vi "Autonomous Independent.vi"() -> ()   [LabVIEW 2016]
doc: "This VI is called when autonomous begins, and will automatically be terminated when autonomous ends. You can carry out timed or sensor driven robot movement independently without needing to return to the caller."
uses:
  <vilib>/Rock Robotics/WPI/ThirdParty/CanMotor/TalonSRX/WPI_CANTalonSRX_APIFeedbackSelect.ctl
  <vilib>/Rock Robotics/WPI/ThirdParty/CanMotor/TalonSRX/WPI_CANTalonSRX_Params.ctl
  <vilib>/Rock Robotics/WPI/ThirdParty/CanMotor/TalonSRX/WPI_CANTalonSRX_APIControlMode.ctl
  <vilib>/Rock Robotics/WPI/Utilities/WPI_GetSetVariantRefNum.vi
  <vilib>/Rock Robotics/Network Tables/NT Read String.vi
  <vilib>/Rock Robotics/Network Tables/NT Write Numeric Array.vi
  <vilib>/Rock Robotics/WPI/RobotDrive/WPI_RobotDriveArcadeDrive_Standard(NoSaturation).vi
  Robot Global Data.vi
panel:
  out "Encoder Position 7":dbl
  out "Encoder Position 6":dbl
  out "RIGHT SIDE":dbl
  out "Encoder Position 4":dbl
  out "Encoder Position 3":dbl
  out "Encoder Position":dbl
  out "Encoder Position 2":dbl
  # "Be sure to right-click and choose Data Operations>>Make Current Value default if you want to save the array values with the VI"
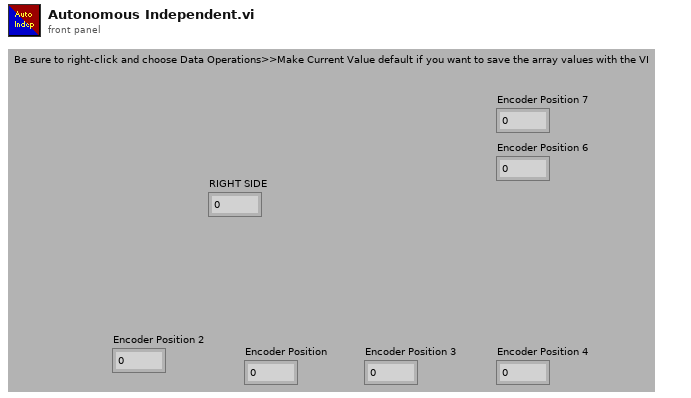
[diagram p1: front panel]
types:
  T1 = typedef "WPI_CANTalonSRX_APIFeedbackSelect.ctl" = enum16{"Digital Quadrature Encoder", "Analog Potentiometer", "Analog Encoder", "Count on Quad-A (Rising-Edge)", "Count on Quad-A (Falling-Edge)", "CTR Magnetic Enc (Absolute)", "CTR Magnetic Enc (Relative)", "Pulse Width"}
  T2 = typedef "WPI_JoystickDevRef.ctl" = cluster{"Device":T3}
  T3 = typedef "WPI_JoystickDeviceEnum.ctl" = enum16{"USB 0", "USB 1", "USB 2", "USB 3", "USB 4", "USB 5"}
  T4 = typedef "WPI_MotorControlDeviceRef.ctl" = cluster{"DeviceStatus":errorcluster, "Type":T5, "PWM":cluster{"PWM Channel":T6, "DeadBand":T7}, "CAN":cluster{"Device Number":u8, "SetOutput VI Ref":variant, "GetOutput VI Ref":variant, "Enable VI Ref":variant, "Disable VI Ref":variant, "Data":variant}, "Invert":bool}
  T5 = typedef "WPI_MotorControlType.ctl" = enum16{"PWM", "CAN"}
  T6 = typedef "FPGA_DIOPWMChannel.ctl" = enum8{"PWM 0", "PWM 1", "PWM 2", "PWM 3", "PWM 4", "PWM 5", "PWM 6", "PWM 7", "PWM 8", "PWM 9", "PWM MXP 0", "PWM MXP 1", "PWM MXP 2", "PWM MXP 3", "PWM MXP 4", "PWM MXP 5", "PWM MXP 6", "PWM MXP 7", "PWM MXP 8", "PWM MXP 9", "Invalid"}
  T7 = typedef "WPI_PWMDeadband.ctl" = cluster{"Name":string, "maxPositivePwm":i32, "minPositivePwm":i32, "centerPwm":i32, "maxNegativePwm":i32, "minNegativePwm":i32, "angularRange":u16}
  T8 = typedef "WPI_RobotDriveDevRef.ctl" = cluster{"DevStatus":errorcluster, "Motors[]":T4[], "Square Inputs":bool, "Max Output":dbl}
  T9 = typedef "WPI_CANTalonSRX_APIControlMode.ctl" = enum8{"Percent VBus", "Speed", "Position", "Slave", "Unchanged / Invalid", "Voltage Compensation", "Current", "Motion Profile", "Motion Magic"}
  T10 = typedef "WPI_CANTalonSRX_Params.ctl" = u8
  T11 = typedef "WPI_CANTalonSRX_GlobalStatus.ctl" = cluster{"Applied Throttle":dbl, "Module Enabled":bool, "CAN Error":errorcluster, "Closed Loop Error":dbl, "Forward Limit Switch Closed":bool, "Reverse Limit Switch Closed":bool, "Sensor Position":dbl, "Sensor Velocity":dbl, "Current":dbl, "Sticky Fault - Over Temp":bool, "Sticky Fault - Under Voltage":bool, "Sticky Fault - Forward Limit":bool, "Sticky Fault - Reverse Limit":bool, "Sticky Fault - Forward Soft Limit":bool, "Sticky Fault - Reverse Soft Limit":bool, "Brake is Enabled":bool, "Encoder Position":dbl, "Encoder Velocity":dbl, "Encoder Index Count":dbl, "Encoder A Pin State":bool, "Encoder B Pin State":bool, "Encoder Index Pin State":bool, "Analog In":dbl, "Analog In Velocity":dbl, "Temperature (C)":dbl, "Battery Voltage":dbl, "Control 5 Is Supported":bool, "Current Profile Slot Select":dbl, "Pos Div 8":bool, "Vel Div 4":bool, "Pulse Width Position":i32, "Pulse Width Velocity":i32, "Pulse Width Rise To Rise (us)":i32, "Pulse Width Rise To Fall (us)":i32, "Mot Prof Active Is Under Run":bool, "Mot Prof Active Has Under Run":bool, "Mot Prof Active Is Last":bool, "Mot Prof Active Velocity Only":bool, "Mot Prof Active Is Valid":bool, "Mot Prof Buffer Is Full":bool, "Mot Prof Active Profile Slot Select":i32, "Mot Prof NextID":i32, "Mot Prof Count":i32, "Mot Prof Active Velocity":dbl, "Mot Prof Active Position":dbl, "Mot Prof Output Enable":i32, "UsageFrame":u32}
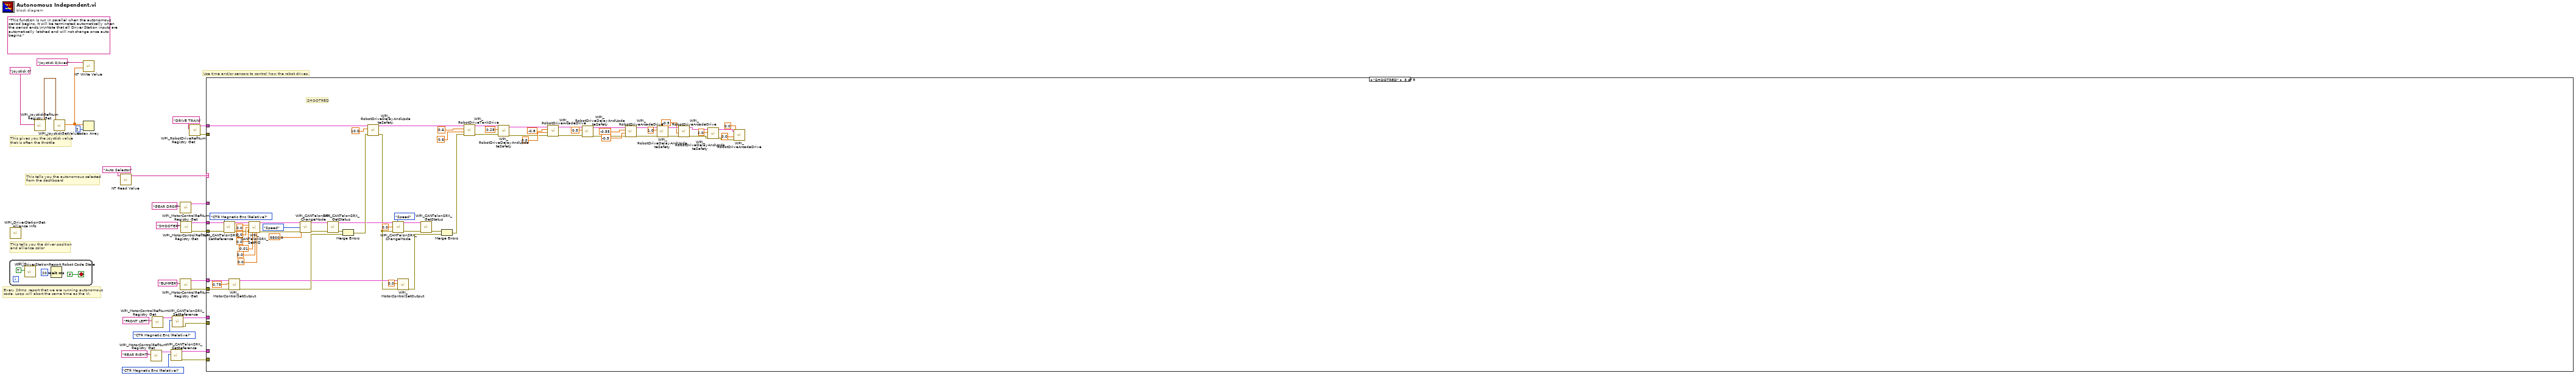
[diagram p0: block diagram]
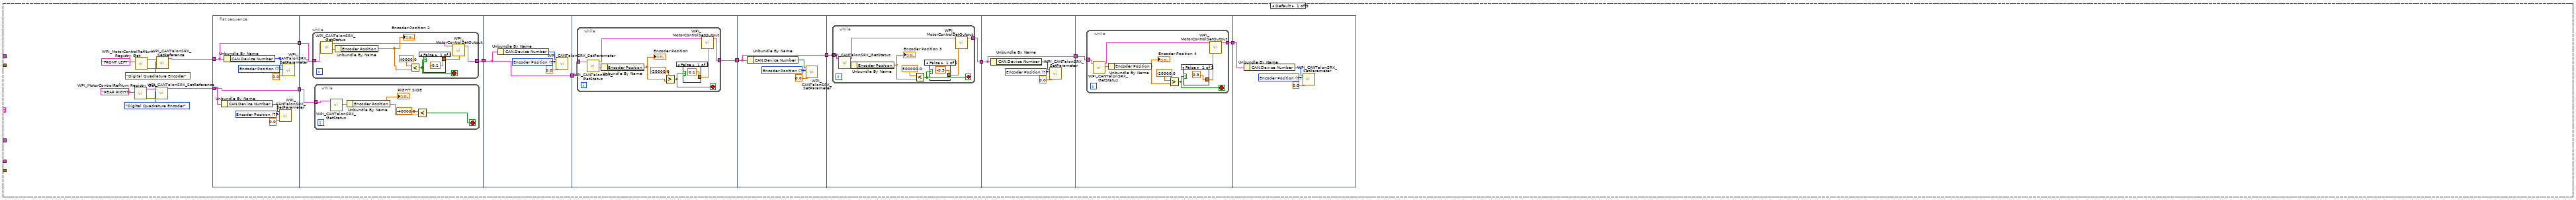
[diagram p2: hidden frame]
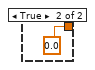
[diagram p3: hidden frame]
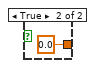
[diagram p4: hidden frame]
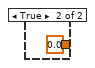
[diagram p5: hidden frame]
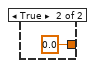
[diagram p6: hidden frame]
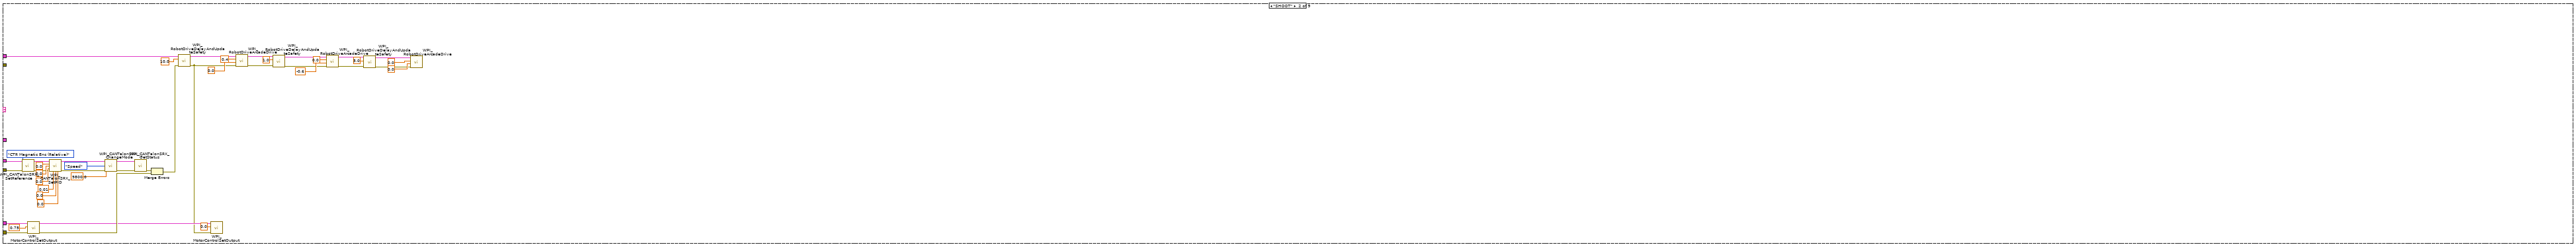
[diagram p7: hidden frame]
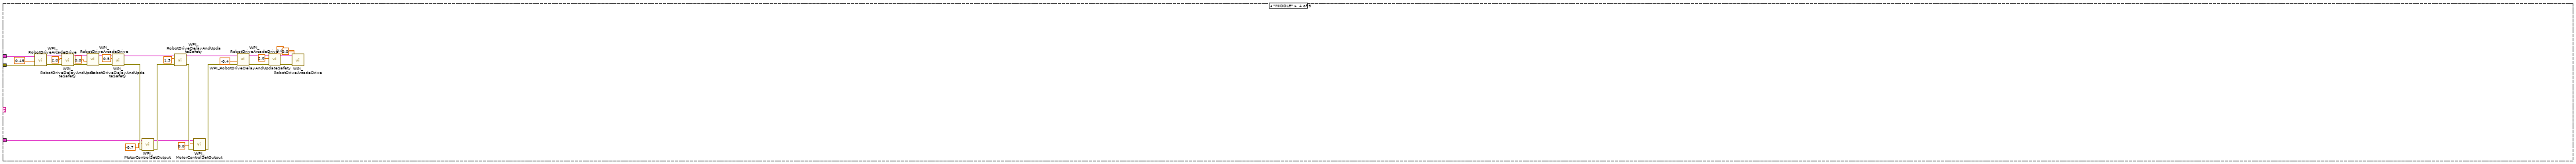
[diagram p8: hidden frame]
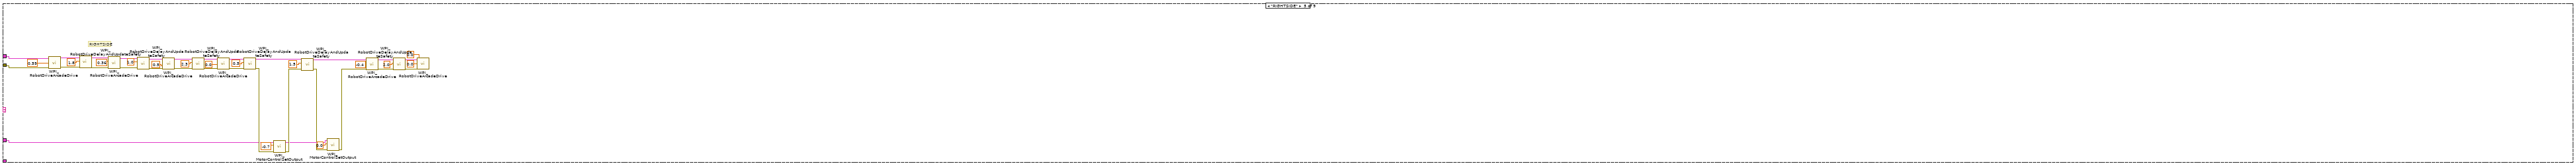
[diagram p9: hidden frame]
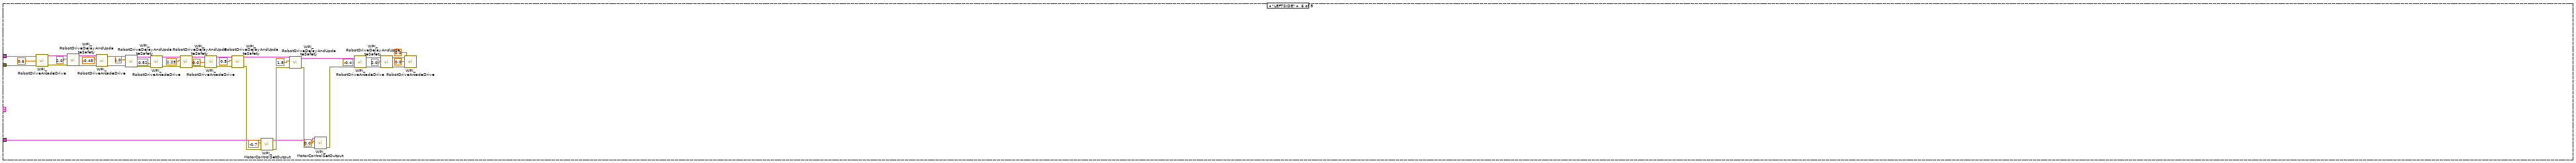
[diagram p10: hidden frame]
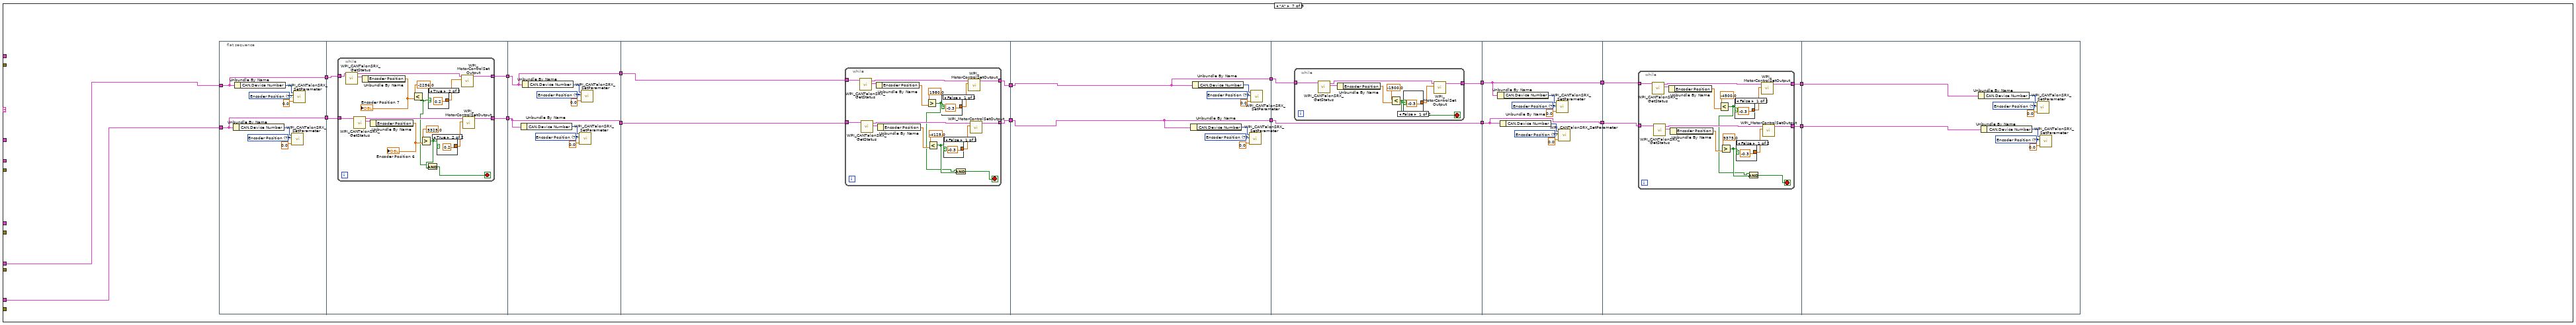
[diagram p11: hidden frame]
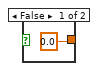
[diagram p12: hidden frame]
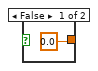
[diagram p13: hidden frame]
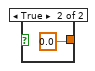
[diagram p14: hidden frame]
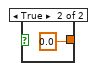
[diagram p15: hidden frame]
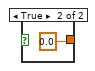
[diagram p16: hidden frame]
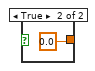
[diagram p17: hidden frame]
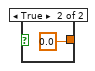
[diagram p18: hidden frame]
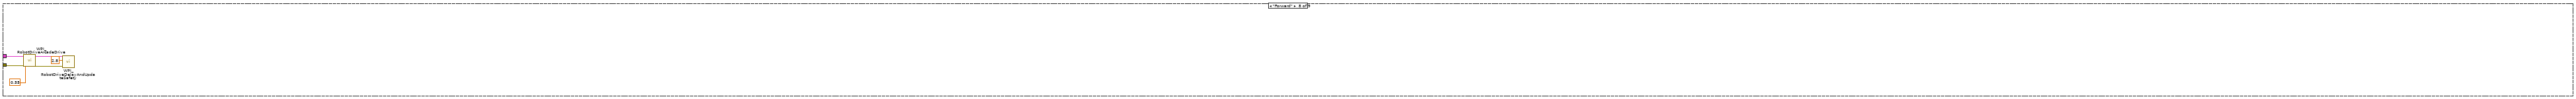
[diagram p19: hidden frame]
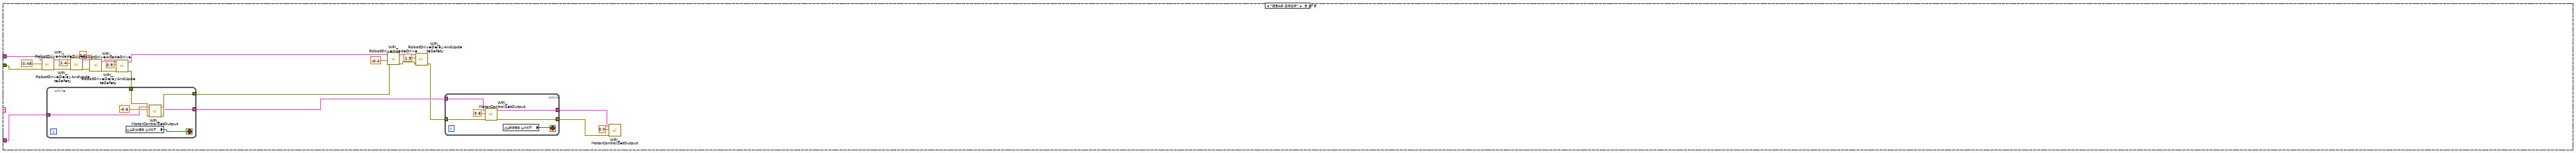
[diagram p20: hidden frame]
diagram:
  (unwired) "This function is run in parallel when the autonomous period begins. It will be terminated automatically when the period ends.\n\nNote that all Driver Station inputs are automatically latched and will not change once auto begins."
  # "Use time and/or sensors to control how the robot drives."
  # "This tells you the autonomous selected\nfrom the dashboard"
  # "Every 20ms, report that we are running autonomous\ncode. Loop will abort the same time as the VI."
  # "This gives you the joystick value\nthat is often the throttle"
  # "This tells you the driver position\nand alliance color"
  n1 = while {
    stop <- FALSE stop-if-true
    n2 = call <vilib>:"WPI_DriverStationReport Robot Code State.vi"("Autonomous"=TRUE) -> ()  [unwired: 10 in, 1 out]
    n3 = Wait (ms)(milliseconds to wait=u32 20) -> ()  [unwired: 1 out]
  }
  n4 = call <vilib>:"WPI_DriverStationGet Alliance Info.vi"() -> ()  [unwired: 12 out]
  n5 = call <vilib>:"WPI_JoystickRefNum Registry Get.vi"("refnum name"="Joystick 0") -> ("JoystickDevRef"=w27:T2)  [unwired: 1 in, 9 out]
  n6 = call <vilib>:"WPI_JoystickGetValues.vi"("JoystickDevRef"=w27) -> ("Axes"=w23:dbl[])  [unwired: 6 in, 4 out]
  n7 = call-poly <vilib>:"NT Write Value.vi"("Numeric Array"=w23, "Name"="Joystick 0/Axes") -> ()  [unwired: 9 in, 1 out]
  n8 = Index Array(array=w23, index=2) -> ()  [unwired: 1 out]
  n9 = call-poly <vilib>:"NT Read Value.vi"("Name"="Auto Selector") -> ("String"=w24:string)  [unwired: 9 in, 1 out]
  n10 = call <vilib>:"WPI_MotorControlRefNum Registry Get.vi"("refnum name"="REAR RIGHT") -> ("MotorControlDevRef"=w17:T4)  [unwired: 9 in, 1 out]
  n11 = call <vilib>:"WPI_MotorControlRefNum Registry Get.vi"("refnum name"="FRONT LEFT") -> ("MotorControlDevRef"=w20:T4)  [unwired: 9 in, 1 out]
  n12 = call <vilib>:"WPI_CANTalonSRX_SetReference.vi"("Feedback Reference"=WPI_CANTalonSRX_APIFeedbackSelect."CTR Magnetic Enc (Relative)", "CAN Talon SRX Ref"=w17) -> ("error out"=w13:errorcluster, "CAN Talon SRX Ref"=w14:T4)  [unwired: 8 in]
  n13 = call <vilib>:"WPI_CANTalonSRX_SetReference.vi"("Feedback Reference"=WPI_CANTalonSRX_APIFeedbackSelect."CTR Magnetic Enc (Relative)", "CAN Talon SRX Ref"=w20) -> ("error out"=w12:errorcluster, "CAN Talon SRX Ref"=w15:T4)  [unwired: 8 in]
  n14 = call <vilib>:"WPI_MotorControlRefNum Registry Get.vi"("refnum name"="GEAR DROP") -> ("MotorControlDevRef"=w7:T4)  [unwired: 9 in, 1 out]
  n15 = call <vilib>:"WPI_MotorControlRefNum Registry Get.vi"("refnum name"="BUMPER") -> ("error out"=w2:errorcluster, "MotorControlDevRef"=w3:T4)  [unwired: 9 in]
  n16 = call <vilib>:"WPI_MotorControlRefNum Registry Get.vi"("refnum name"="SHOOTER") -> ("error out"=w4:errorcluster, "MotorControlDevRef"=w5:T4)  [unwired: 9 in]
  n17 = call <vilib>:"WPI_RobotDriveRefNum Registry Get.vi"("refnum name"="DRIVE TRAIN") -> ("error out"=w9:errorcluster, "RobotDriveDevRef"=w10:T8)  [unwired: 9 in]
  n18 = case shown="\"SHOOTRED\"" w24 {
    tunnel: w15 -> [_ _ _ _ _ _ w362 _ _]
    tunnel: w14 -> [_ _ _ _ _ _ w361 _ _]
    tunnel: w13 -> [_ _ _ _ _ _ _ _ _]
    tunnel: w12 -> [_ _ _ _ _ _ _ _ _]
    tunnel: w10 -> [_ w155 w221 w270 w273 w356 _ w508 w533]
    tunnel: w9 -> [_ _ _ w269 w272 w355 _ w507 w532]
    tunnel: w7 -> [_ _ _ w257 w271 w332 _ _ w513]
    tunnel: w5 -> [_ w161 w227 _ _ _ _ _ _]
    tunnel: w4 -> [_ w160 w226 _ _ _ _ _ _]
    tunnel: w3 -> [_ w146 w214 _ _ _ _ _ _]
    tunnel: w2 -> [_ w145 w213 _ _ _ _ _ _]
    frame Default {
      n19 = call <vilib>:"WPI_MotorControlRefNum Registry Get.vi"("refnum name"="REAR RIGHT") -> ("error out"=w36:errorcluster, "MotorControlDevRef"=w35:T4)  [unwired: 9 in]
      n20 = call <vilib>:"WPI_MotorControlRefNum Registry Get.vi"("refnum name"="FRONT LEFT") -> ("error out"=w48:errorcluster, "MotorControlDevRef"=w49:T4)  [unwired: 9 in]
      n21 = call <vilib>:"WPI_CANTalonSRX_SetReference.vi"("error in (no error)"=w36, "Feedback Reference"=WPI_CANTalonSRX_APIFeedbackSelect."Digital Quadrature Encoder", "CAN Talon SRX Ref"=w35) -> ("CAN Talon SRX Ref"=w33:T4)  [unwired: 7 in, 1 out]
      n22 = call <vilib>:"WPI_CANTalonSRX_SetReference.vi"("error in (no error)"=w48, "Feedback Reference"=WPI_CANTalonSRX_APIFeedbackSelect."Digital Quadrature Encoder", "CAN Talon SRX Ref"=w49) -> ("CAN Talon SRX Ref"=w44:T4)  [unwired: 7 in, 1 out]
      n23 = flat-sequence {
        tunnel: w44 -> [w55]
        tunnel: [w55] -> w43
        tunnel: w33 -> [w51]
        tunnel: [w51] -> w32
        tunnel: [w60] -> w46
        tunnel: w43 -> [w61]
        tunnel: w32 -> [w59]
        tunnel: w46 -> [w77]
        tunnel: [w77] -> w45
        tunnel: w45 -> [w82]
        tunnel: [w81] -> w42
        tunnel: w42 -> [w93]
        tunnel: [w93] -> w41
        tunnel: w41 -> [w98]
        tunnel: [w97] -> w40
        tunnel: w40 -> [w109]
        tunnel: [w109] -> w39
        tunnel: w39 -> [w114]
        tunnel: [w113] -> w38
        tunnel: w38 -> [w125]
        frame #0 {
          w53 = T10 77 items=["Slot 0 - P"=1, "Slot 0 - I"=2, "Slot 0 - D"=3, "Slot 0 - F"=4, "Slot 0 - I Zone"=5, "Slot 0 - Ramp Rate"=6, "Slot 1 - P"=11, "Slot 1 - I"=12, "Slot 1 - D"=13, "Slot 1 - F"=14, "Slot 1 - I Zone"=15, "Slot 1 - Ramp Rate"=16, "Soft Limit - Forward"=21, "Soft Limit - Reverse"=22, "Soft Limit - Forward Enable"=23, "Soft Limit - Reverse Enable"=24, "On Boot - Brake Mode"=31, "On Boot - Limit Normally Closed - Forward"=32, "On Boot - Limit Normally Closed - Reverse"=33, "On Boot - Limit Disabled - Forward"=34, "On Boot - Limit Disabled - Reverse"=35, "Fault - Over Temp"=41, "Fault - Under Voltage"=42, "Fault - Forward Limit"=43, "Fault - Reverse Limit"=44, "Fault - Hardware Failure"=45, "Fault - Forward Soft Limit"=46, "Fault - Reverse Soft Limit"=47, "Sticky Fault - Over Temp"=48, "Sticky Fault - Under Voltage"=49, "Sticky Fault - Forward Limit"=50, "Sticky Fault - Reverse Limit"=51, "Sticky Fault - Forward Soft Limit"=52, "Sticky Fault - Reverse Soft Limit"=53, "Applied Throttle"=61, "Closed-Loop Error"=62, "Select Feedback Device"=63, "Reverse Closed-Loop Output"=64, "Mode Select"=65, "Profile Slot Select"=66, "Ramp Throttle"=67, "Reverse Feedback Sensor"=68, "Limit Switch Enabled"=69, "Limit Switch Closed - Forward"=70, "Limit Switch Closed - Reverse"=71, "Sensor Position"=73, "Sensor Velocity"=74, "Current"=75, "Brake is Enabled"=76, "Encoder Position"=77, "Encoder Velocity"=78, "Encoder Index Rise Events"=79, "Encoder A Pin State"=80, "Encoder B Pin State"=81, "Encoder Index Pin State"=82, "Analog In with Overflow"=83, "Analog In Velocity"=84, "Temperature"=85, "Battery Voltage"=86, "Reset Count"=87, "Reset Flags"=88, "Firmware Version"=89, "Settings Changed"=90, "Quad Filter Enable"=91, "Ignore Disable Broadcast"=92, "I Accumulator"=93, "Status 1 Frame Rate Ms"=94, "Status 2 Frame Rate Ms"=95, "Status 3 Frame Rate Ms"=96, "Status 4 Frame Rate Ms"=97, "Status 6 Frame Rate Ms"=98, "Status 7 Frame Rate Ms"=99, "Enable Index Pin Clear Position"=100, "Peak Positive Output"=104, "Nominal Positive Output"=105, "Peak Negative Output"=106, "Nominal Negative Output"=107, "Quad Index Pin Polarity"=108, "Status 8 Frame Rate Ms"=109, "Allow Position Overflow"=110, "Slot 0 - Allowable Closed-Loop Error"=111, "Number Potentiometer Turns"=112, "Encoder Codes Per Rev"=113, "Pulse Width Decoded Position"=114, "Analog Position"=115, "Voltage Compensation Rate (V/s)"=116, "Slot 1 - Allowable Closed-Loop Error"=117, "Motion Profile Has Underrun Err"=119, "Reserved 120"=120, "Legacy Control Mode"=121, "Motion Magic Acceleration"=122, "Motion Magic Cruise Velocity"=123, "Status 10 Frame Rate"=124, "Current Limit Threshold"=125, "CustomParam0"=137, "CustomParam1"=138, "PersStorageSaving"=139, "ClearPositionOnLimitF"=144, "ClearPositionOnLimitR"=145, "NominalBatteryVoltage"=146, "SampleVelocityPeriod"=147, "SampleVelocityWindow"=148] ("Parameter")
          w57 = T10 77 items=["Slot 0 - P"=1, "Slot 0 - I"=2, "Slot 0 - D"=3, "Slot 0 - F"=4, "Slot 0 - I Zone"=5, "Slot 0 - Ramp Rate"=6, "Slot 1 - P"=11, "Slot 1 - I"=12, "Slot 1 - D"=13, "Slot 1 - F"=14, "Slot 1 - I Zone"=15, "Slot 1 - Ramp Rate"=16, "Soft Limit - Forward"=21, "Soft Limit - Reverse"=22, "Soft Limit - Forward Enable"=23, "Soft Limit - Reverse Enable"=24, "On Boot - Brake Mode"=31, "On Boot - Limit Normally Closed - Forward"=32, "On Boot - Limit Normally Closed - Reverse"=33, "On Boot - Limit Disabled - Forward"=34, "On Boot - Limit Disabled - Reverse"=35, "Fault - Over Temp"=41, "Fault - Under Voltage"=42, "Fault - Forward Limit"=43, "Fault - Reverse Limit"=44, "Fault - Hardware Failure"=45, "Fault - Forward Soft Limit"=46, "Fault - Reverse Soft Limit"=47, "Sticky Fault - Over Temp"=48, "Sticky Fault - Under Voltage"=49, "Sticky Fault - Forward Limit"=50, "Sticky Fault - Reverse Limit"=51, "Sticky Fault - Forward Soft Limit"=52, "Sticky Fault - Reverse Soft Limit"=53, "Applied Throttle"=61, "Closed-Loop Error"=62, "Select Feedback Device"=63, "Reverse Closed-Loop Output"=64, "Mode Select"=65, "Profile Slot Select"=66, "Ramp Throttle"=67, "Reverse Feedback Sensor"=68, "Limit Switch Enabled"=69, "Limit Switch Closed - Forward"=70, "Limit Switch Closed - Reverse"=71, "Sensor Position"=73, "Sensor Velocity"=74, "Current"=75, "Brake is Enabled"=76, "Encoder Position"=77, "Encoder Velocity"=78, "Encoder Index Rise Events"=79, "Encoder A Pin State"=80, "Encoder B Pin State"=81, "Encoder Index Pin State"=82, "Analog In with Overflow"=83, "Analog In Velocity"=84, "Temperature"=85, "Battery Voltage"=86, "Reset Count"=87, "Reset Flags"=88, "Firmware Version"=89, "Settings Changed"=90, "Quad Filter Enable"=91, "Ignore Disable Broadcast"=92, "I Accumulator"=93, "Status 1 Frame Rate Ms"=94, "Status 2 Frame Rate Ms"=95, "Status 3 Frame Rate Ms"=96, "Status 4 Frame Rate Ms"=97, "Status 6 Frame Rate Ms"=98, "Status 7 Frame Rate Ms"=99, "Enable Index Pin Clear Position"=100, "Peak Positive Output"=104, "Nominal Positive Output"=105, "Peak Negative Output"=106, "Nominal Negative Output"=107, "Quad Index Pin Polarity"=108, "Status 8 Frame Rate Ms"=109, "Allow Position Overflow"=110, "Slot 0 - Allowable Closed-Loop Error"=111, "Number Potentiometer Turns"=112, "Encoder Codes Per Rev"=113, "Pulse Width Decoded Position"=114, "Analog Position"=115, "Voltage Compensation Rate (V/s)"=116, "Slot 1 - Allowable Closed-Loop Error"=117, "Motion Profile Has Underrun Err"=119, "Reserved 120"=120, "Legacy Control Mode"=121, "Motion Magic Acceleration"=122, "Motion Magic Cruise Velocity"=123, "Status 10 Frame Rate"=124, "Current Limit Threshold"=125, "CustomParam0"=137, "CustomParam1"=138, "PersStorageSaving"=139, "ClearPositionOnLimitF"=144, "ClearPositionOnLimitR"=145, "NominalBatteryVoltage"=146, "SampleVelocityPeriod"=147, "SampleVelocityWindow"=148] ("Parameter")
          n24 = Unbundle By Name(w51) -> ("CAN.Device Number"=w52:u8)
          n25 = Unbundle By Name(w55) -> ("CAN.Device Number"=w58:u8)
          n26 = call <vilib>:"WPI_CANTalonSRX_SetParameter.vi"("Value"=0.0, "Parameter"=w53, "Device ID (0)"=w52) -> ()  [unwired: 7 in, 2 out]
          n27 = call <vilib>:"WPI_CANTalonSRX_SetParameter.vi"("Value"=0.0, "Parameter"=w57, "Device ID (0)"=w58) -> ()  [unwired: 7 in, 2 out]
        }
        frame #1 {
          n28 = while {
            tunnel: w61 -> [w68]
            tunnel: [w67] -> w60
            stop <- w71 stop-if-true
            n29 = call <vilib>:"WPI_CANTalonSRX_GetStatus.vi"("CAN Talon SRX Ref"=w68) -> ("Talon SRX Status"=w74:T11, "CAN Talon SRX Ref"=w73:T4)  [unwired: 8 in, 1 out]
            n30 = Unbundle By Name(w74) -> ("Encoder Position"=w70:dbl)
            "Encoder Position 2" <- w70
            n31 = Less?(x=40000.0, y=w70) -> (x < y?=w71:bool)
            n32 = case shown="False" w71 {
              tunnel: [-0.1 ("x") 0.0 ("x")] -> w72
              frame False {
              }
              frame True {
              }
            }
            n33 = call <vilib>:"WPI_MotorControlSetOutput.vi"("Output"=w72, "MotorControlDevRef"=w73) -> ("MotorControlDevRef"=w67:T4)  [unwired: 7 in, 2 out]
          }
          n34 = while {
            tunnel: w59 -> [w66]
            stop <- w63 stop-if-true
            n35 = call <vilib>:"WPI_CANTalonSRX_GetStatus.vi"("CAN Talon SRX Ref"=w66) -> ("Talon SRX Status"=w62:T11)  [unwired: 8 in, 2 out]
            n36 = Unbundle By Name(w62) -> ("Encoder Position"=w65:dbl)
            "RIGHT SIDE" <- w65
            n37 = Less?(x=-40000.0, y=w65) -> (x < y?=w63:bool)
          }
        }
        frame #2 {
          w79 = T10 77 items=["Slot 0 - P"=1, "Slot 0 - I"=2, "Slot 0 - D"=3, "Slot 0 - F"=4, "Slot 0 - I Zone"=5, "Slot 0 - Ramp Rate"=6, "Slot 1 - P"=11, "Slot 1 - I"=12, "Slot 1 - D"=13, "Slot 1 - F"=14, "Slot 1 - I Zone"=15, "Slot 1 - Ramp Rate"=16, "Soft Limit - Forward"=21, "Soft Limit - Reverse"=22, "Soft Limit - Forward Enable"=23, "Soft Limit - Reverse Enable"=24, "On Boot - Brake Mode"=31, "On Boot - Limit Normally Closed - Forward"=32, "On Boot - Limit Normally Closed - Reverse"=33, "On Boot - Limit Disabled - Forward"=34, "On Boot - Limit Disabled - Reverse"=35, "Fault - Over Temp"=41, "Fault - Under Voltage"=42, "Fault - Forward Limit"=43, "Fault - Reverse Limit"=44, "Fault - Hardware Failure"=45, "Fault - Forward Soft Limit"=46, "Fault - Reverse Soft Limit"=47, "Sticky Fault - Over Temp"=48, "Sticky Fault - Under Voltage"=49, "Sticky Fault - Forward Limit"=50, "Sticky Fault - Reverse Limit"=51, "Sticky Fault - Forward Soft Limit"=52, "Sticky Fault - Reverse Soft Limit"=53, "Applied Throttle"=61, "Closed-Loop Error"=62, "Select Feedback Device"=63, "Reverse Closed-Loop Output"=64, "Mode Select"=65, "Profile Slot Select"=66, "Ramp Throttle"=67, "Reverse Feedback Sensor"=68, "Limit Switch Enabled"=69, "Limit Switch Closed - Forward"=70, "Limit Switch Closed - Reverse"=71, "Sensor Position"=73, "Sensor Velocity"=74, "Current"=75, "Brake is Enabled"=76, "Encoder Position"=77, "Encoder Velocity"=78, "Encoder Index Rise Events"=79, "Encoder A Pin State"=80, "Encoder B Pin State"=81, "Encoder Index Pin State"=82, "Analog In with Overflow"=83, "Analog In Velocity"=84, "Temperature"=85, "Battery Voltage"=86, "Reset Count"=87, "Reset Flags"=88, "Firmware Version"=89, "Settings Changed"=90, "Quad Filter Enable"=91, "Ignore Disable Broadcast"=92, "I Accumulator"=93, "Status 1 Frame Rate Ms"=94, "Status 2 Frame Rate Ms"=95, "Status 3 Frame Rate Ms"=96, "Status 4 Frame Rate Ms"=97, "Status 6 Frame Rate Ms"=98, "Status 7 Frame Rate Ms"=99, "Enable Index Pin Clear Position"=100, "Peak Positive Output"=104, "Nominal Positive Output"=105, "Peak Negative Output"=106, "Nominal Negative Output"=107, "Quad Index Pin Polarity"=108, "Status 8 Frame Rate Ms"=109, "Allow Position Overflow"=110, "Slot 0 - Allowable Closed-Loop Error"=111, "Number Potentiometer Turns"=112, "Encoder Codes Per Rev"=113, "Pulse Width Decoded Position"=114, "Analog Position"=115, "Voltage Compensation Rate (V/s)"=116, "Slot 1 - Allowable Closed-Loop Error"=117, "Motion Profile Has Underrun Err"=119, "Reserved 120"=120, "Legacy Control Mode"=121, "Motion Magic Acceleration"=122, "Motion Magic Cruise Velocity"=123, "Status 10 Frame Rate"=124, "Current Limit Threshold"=125, "CustomParam0"=137, "CustomParam1"=138, "PersStorageSaving"=139, "ClearPositionOnLimitF"=144, "ClearPositionOnLimitR"=145, "NominalBatteryVoltage"=146, "SampleVelocityPeriod"=147, "SampleVelocityWindow"=148] ("Parameter")
          n38 = Unbundle By Name(w77) -> ("CAN.Device Number"=w80:u8)
          n39 = call <vilib>:"WPI_CANTalonSRX_SetParameter.vi"("Value"=0.0, "Parameter"=w79, "Device ID (0)"=w80) -> ()  [unwired: 7 in, 2 out]
        }
        frame #3 {
          n40 = while {
            tunnel: w82 -> [w84]
            tunnel: [w83] -> w81
            stop <- w87 stop-if-true
            n41 = call <vilib>:"WPI_CANTalonSRX_GetStatus.vi"("CAN Talon SRX Ref"=w84) -> ("Talon SRX Status"=w90:T11, "CAN Talon SRX Ref"=w89:T4)  [unwired: 8 in, 1 out]
            n42 = Unbundle By Name(w90) -> ("Encoder Position"=w86:dbl)
            "Encoder Position" <- w86
            n43 = Greater?(x=-20000.0 ("y"), y=w86) -> (0:w87:bool)
            n44 = case shown="False" w87 {
              tunnel: [0.1 ("x") 0.0 ("x")] -> w88
              frame False {
              }
              frame True {
              }
            }
            n45 = call <vilib>:"WPI_MotorControlSetOutput.vi"("Output"=w88, "MotorControlDevRef"=w89) -> ("MotorControlDevRef"=w83:T4)  [unwired: 7 in, 2 out]
          }
        }
        frame #4 {
          w95 = T10 77 items=["Slot 0 - P"=1, "Slot 0 - I"=2, "Slot 0 - D"=3, "Slot 0 - F"=4, "Slot 0 - I Zone"=5, "Slot 0 - Ramp Rate"=6, "Slot 1 - P"=11, "Slot 1 - I"=12, "Slot 1 - D"=13, "Slot 1 - F"=14, "Slot 1 - I Zone"=15, "Slot 1 - Ramp Rate"=16, "Soft Limit - Forward"=21, "Soft Limit - Reverse"=22, "Soft Limit - Forward Enable"=23, "Soft Limit - Reverse Enable"=24, "On Boot - Brake Mode"=31, "On Boot - Limit Normally Closed - Forward"=32, "On Boot - Limit Normally Closed - Reverse"=33, "On Boot - Limit Disabled - Forward"=34, "On Boot - Limit Disabled - Reverse"=35, "Fault - Over Temp"=41, "Fault - Under Voltage"=42, "Fault - Forward Limit"=43, "Fault - Reverse Limit"=44, "Fault - Hardware Failure"=45, "Fault - Forward Soft Limit"=46, "Fault - Reverse Soft Limit"=47, "Sticky Fault - Over Temp"=48, "Sticky Fault - Under Voltage"=49, "Sticky Fault - Forward Limit"=50, "Sticky Fault - Reverse Limit"=51, "Sticky Fault - Forward Soft Limit"=52, "Sticky Fault - Reverse Soft Limit"=53, "Applied Throttle"=61, "Closed-Loop Error"=62, "Select Feedback Device"=63, "Reverse Closed-Loop Output"=64, "Mode Select"=65, "Profile Slot Select"=66, "Ramp Throttle"=67, "Reverse Feedback Sensor"=68, "Limit Switch Enabled"=69, "Limit Switch Closed - Forward"=70, "Limit Switch Closed - Reverse"=71, "Sensor Position"=73, "Sensor Velocity"=74, "Current"=75, "Brake is Enabled"=76, "Encoder Position"=77, "Encoder Velocity"=78, "Encoder Index Rise Events"=79, "Encoder A Pin State"=80, "Encoder B Pin State"=81, "Encoder Index Pin State"=82, "Analog In with Overflow"=83, "Analog In Velocity"=84, "Temperature"=85, "Battery Voltage"=86, "Reset Count"=87, "Reset Flags"=88, "Firmware Version"=89, "Settings Changed"=90, "Quad Filter Enable"=91, "Ignore Disable Broadcast"=92, "I Accumulator"=93, "Status 1 Frame Rate Ms"=94, "Status 2 Frame Rate Ms"=95, "Status 3 Frame Rate Ms"=96, "Status 4 Frame Rate Ms"=97, "Status 6 Frame Rate Ms"=98, "Status 7 Frame Rate Ms"=99, "Enable Index Pin Clear Position"=100, "Peak Positive Output"=104, "Nominal Positive Output"=105, "Peak Negative Output"=106, "Nominal Negative Output"=107, "Quad Index Pin Polarity"=108, "Status 8 Frame Rate Ms"=109, "Allow Position Overflow"=110, "Slot 0 - Allowable Closed-Loop Error"=111, "Number Potentiometer Turns"=112, "Encoder Codes Per Rev"=113, "Pulse Width Decoded Position"=114, "Analog Position"=115, "Voltage Compensation Rate (V/s)"=116, "Slot 1 - Allowable Closed-Loop Error"=117, "Motion Profile Has Underrun Err"=119, "Reserved 120"=120, "Legacy Control Mode"=121, "Motion Magic Acceleration"=122, "Motion Magic Cruise Velocity"=123, "Status 10 Frame Rate"=124, "Current Limit Threshold"=125, "CustomParam0"=137, "CustomParam1"=138, "PersStorageSaving"=139, "ClearPositionOnLimitF"=144, "ClearPositionOnLimitR"=145, "NominalBatteryVoltage"=146, "SampleVelocityPeriod"=147, "SampleVelocityWindow"=148] ("Parameter")
          n46 = Unbundle By Name(w93) -> ("CAN.Device Number"=w96:u8)
          n47 = call <vilib>:"WPI_CANTalonSRX_SetParameter.vi"("Value"=0.0, "Parameter"=w95, "Device ID (0)"=w96) -> ()  [unwired: 7 in, 2 out]
        }
        frame #5 {
          n48 = while {
            tunnel: w98 -> [w100]
            tunnel: [w99] -> w97
            stop <- w103 stop-if-true
            n49 = call <vilib>:"WPI_CANTalonSRX_GetStatus.vi"("CAN Talon SRX Ref"=w100) -> ("Talon SRX Status"=w106:T11, "CAN Talon SRX Ref"=w105:T4)  [unwired: 8 in, 1 out]
            n50 = Unbundle By Name(w106) -> ("Encoder Position"=w102:dbl)
            "Encoder Position 3" <- w102
            n51 = Less?(x=500000.0, y=w102) -> (x < y?=w103:bool)
            n52 = case shown="False" w103 {
              tunnel: [-0.5 ("x") 0.0 ("x")] -> w104
              frame False {
              }
              frame True {
              }
            }
            n53 = call <vilib>:"WPI_MotorControlSetOutput.vi"("Output"=w104, "MotorControlDevRef"=w105) -> ("MotorControlDevRef"=w99:T4)  [unwired: 7 in, 2 out]
          }
        }
        frame #6 {
          w111 = T10 77 items=["Slot 0 - P"=1, "Slot 0 - I"=2, "Slot 0 - D"=3, "Slot 0 - F"=4, "Slot 0 - I Zone"=5, "Slot 0 - Ramp Rate"=6, "Slot 1 - P"=11, "Slot 1 - I"=12, "Slot 1 - D"=13, "Slot 1 - F"=14, "Slot 1 - I Zone"=15, "Slot 1 - Ramp Rate"=16, "Soft Limit - Forward"=21, "Soft Limit - Reverse"=22, "Soft Limit - Forward Enable"=23, "Soft Limit - Reverse Enable"=24, "On Boot - Brake Mode"=31, "On Boot - Limit Normally Closed - Forward"=32, "On Boot - Limit Normally Closed - Reverse"=33, "On Boot - Limit Disabled - Forward"=34, "On Boot - Limit Disabled - Reverse"=35, "Fault - Over Temp"=41, "Fault - Under Voltage"=42, "Fault - Forward Limit"=43, "Fault - Reverse Limit"=44, "Fault - Hardware Failure"=45, "Fault - Forward Soft Limit"=46, "Fault - Reverse Soft Limit"=47, "Sticky Fault - Over Temp"=48, "Sticky Fault - Under Voltage"=49, "Sticky Fault - Forward Limit"=50, "Sticky Fault - Reverse Limit"=51, "Sticky Fault - Forward Soft Limit"=52, "Sticky Fault - Reverse Soft Limit"=53, "Applied Throttle"=61, "Closed-Loop Error"=62, "Select Feedback Device"=63, "Reverse Closed-Loop Output"=64, "Mode Select"=65, "Profile Slot Select"=66, "Ramp Throttle"=67, "Reverse Feedback Sensor"=68, "Limit Switch Enabled"=69, "Limit Switch Closed - Forward"=70, "Limit Switch Closed - Reverse"=71, "Sensor Position"=73, "Sensor Velocity"=74, "Current"=75, "Brake is Enabled"=76, "Encoder Position"=77, "Encoder Velocity"=78, "Encoder Index Rise Events"=79, "Encoder A Pin State"=80, "Encoder B Pin State"=81, "Encoder Index Pin State"=82, "Analog In with Overflow"=83, "Analog In Velocity"=84, "Temperature"=85, "Battery Voltage"=86, "Reset Count"=87, "Reset Flags"=88, "Firmware Version"=89, "Settings Changed"=90, "Quad Filter Enable"=91, "Ignore Disable Broadcast"=92, "I Accumulator"=93, "Status 1 Frame Rate Ms"=94, "Status 2 Frame Rate Ms"=95, "Status 3 Frame Rate Ms"=96, "Status 4 Frame Rate Ms"=97, "Status 6 Frame Rate Ms"=98, "Status 7 Frame Rate Ms"=99, "Enable Index Pin Clear Position"=100, "Peak Positive Output"=104, "Nominal Positive Output"=105, "Peak Negative Output"=106, "Nominal Negative Output"=107, "Quad Index Pin Polarity"=108, "Status 8 Frame Rate Ms"=109, "Allow Position Overflow"=110, "Slot 0 - Allowable Closed-Loop Error"=111, "Number Potentiometer Turns"=112, "Encoder Codes Per Rev"=113, "Pulse Width Decoded Position"=114, "Analog Position"=115, "Voltage Compensation Rate (V/s)"=116, "Slot 1 - Allowable Closed-Loop Error"=117, "Motion Profile Has Underrun Err"=119, "Reserved 120"=120, "Legacy Control Mode"=121, "Motion Magic Acceleration"=122, "Motion Magic Cruise Velocity"=123, "Status 10 Frame Rate"=124, "Current Limit Threshold"=125, "CustomParam0"=137, "CustomParam1"=138, "PersStorageSaving"=139, "ClearPositionOnLimitF"=144, "ClearPositionOnLimitR"=145, "NominalBatteryVoltage"=146, "SampleVelocityPeriod"=147, "SampleVelocityWindow"=148] ("Parameter")
          n54 = Unbundle By Name(w109) -> ("CAN.Device Number"=w110:u8)
          n55 = call <vilib>:"WPI_CANTalonSRX_SetParameter.vi"("Value"=0.0, "Parameter"=w111, "Device ID (0)"=w110) -> ()  [unwired: 7 in, 2 out]
        }
        frame #7 {
          n56 = while {
            tunnel: w114 -> [w116]
            tunnel: [w115] -> w113
            stop <- w119 stop-if-true
            n57 = call <vilib>:"WPI_CANTalonSRX_GetStatus.vi"("CAN Talon SRX Ref"=w116) -> ("Talon SRX Status"=w122:T11, "CAN Talon SRX Ref"=w121:T4)  [unwired: 8 in, 1 out]
            n58 = Unbundle By Name(w122) -> ("Encoder Position"=w118:dbl)
            "Encoder Position 4" <- w118
            n59 = Greater?(x=-20000.0, y=w118) -> (0:w119:bool)
            n60 = case shown="False" w119 {
              tunnel: [0.3 ("x") 0.0 ("x")] -> w120
              frame False {
              }
              frame True {
              }
            }
            n61 = call <vilib>:"WPI_MotorControlSetOutput.vi"("Output"=w120, "MotorControlDevRef"=w121) -> ("MotorControlDevRef"=w115:T4)  [unwired: 7 in, 2 out]
          }
        }
        frame #8 {
          w127 = T10 77 items=["Slot 0 - P"=1, "Slot 0 - I"=2, "Slot 0 - D"=3, "Slot 0 - F"=4, "Slot 0 - I Zone"=5, "Slot 0 - Ramp Rate"=6, "Slot 1 - P"=11, "Slot 1 - I"=12, "Slot 1 - D"=13, "Slot 1 - F"=14, "Slot 1 - I Zone"=15, "Slot 1 - Ramp Rate"=16, "Soft Limit - Forward"=21, "Soft Limit - Reverse"=22, "Soft Limit - Forward Enable"=23, "Soft Limit - Reverse Enable"=24, "On Boot - Brake Mode"=31, "On Boot - Limit Normally Closed - Forward"=32, "On Boot - Limit Normally Closed - Reverse"=33, "On Boot - Limit Disabled - Forward"=34, "On Boot - Limit Disabled - Reverse"=35, "Fault - Over Temp"=41, "Fault - Under Voltage"=42, "Fault - Forward Limit"=43, "Fault - Reverse Limit"=44, "Fault - Hardware Failure"=45, "Fault - Forward Soft Limit"=46, "Fault - Reverse Soft Limit"=47, "Sticky Fault - Over Temp"=48, "Sticky Fault - Under Voltage"=49, "Sticky Fault - Forward Limit"=50, "Sticky Fault - Reverse Limit"=51, "Sticky Fault - Forward Soft Limit"=52, "Sticky Fault - Reverse Soft Limit"=53, "Applied Throttle"=61, "Closed-Loop Error"=62, "Select Feedback Device"=63, "Reverse Closed-Loop Output"=64, "Mode Select"=65, "Profile Slot Select"=66, "Ramp Throttle"=67, "Reverse Feedback Sensor"=68, "Limit Switch Enabled"=69, "Limit Switch Closed - Forward"=70, "Limit Switch Closed - Reverse"=71, "Sensor Position"=73, "Sensor Velocity"=74, "Current"=75, "Brake is Enabled"=76, "Encoder Position"=77, "Encoder Velocity"=78, "Encoder Index Rise Events"=79, "Encoder A Pin State"=80, "Encoder B Pin State"=81, "Encoder Index Pin State"=82, "Analog In with Overflow"=83, "Analog In Velocity"=84, "Temperature"=85, "Battery Voltage"=86, "Reset Count"=87, "Reset Flags"=88, "Firmware Version"=89, "Settings Changed"=90, "Quad Filter Enable"=91, "Ignore Disable Broadcast"=92, "I Accumulator"=93, "Status 1 Frame Rate Ms"=94, "Status 2 Frame Rate Ms"=95, "Status 3 Frame Rate Ms"=96, "Status 4 Frame Rate Ms"=97, "Status 6 Frame Rate Ms"=98, "Status 7 Frame Rate Ms"=99, "Enable Index Pin Clear Position"=100, "Peak Positive Output"=104, "Nominal Positive Output"=105, "Peak Negative Output"=106, "Nominal Negative Output"=107, "Quad Index Pin Polarity"=108, "Status 8 Frame Rate Ms"=109, "Allow Position Overflow"=110, "Slot 0 - Allowable Closed-Loop Error"=111, "Number Potentiometer Turns"=112, "Encoder Codes Per Rev"=113, "Pulse Width Decoded Position"=114, "Analog Position"=115, "Voltage Compensation Rate (V/s)"=116, "Slot 1 - Allowable Closed-Loop Error"=117, "Motion Profile Has Underrun Err"=119, "Reserved 120"=120, "Legacy Control Mode"=121, "Motion Magic Acceleration"=122, "Motion Magic Cruise Velocity"=123, "Status 10 Frame Rate"=124, "Current Limit Threshold"=125, "CustomParam0"=137, "CustomParam1"=138, "PersStorageSaving"=139, "ClearPositionOnLimitF"=144, "ClearPositionOnLimitR"=145, "NominalBatteryVoltage"=146, "SampleVelocityPeriod"=147, "SampleVelocityWindow"=148] ("Parameter")
          n62 = Unbundle By Name(w125) -> ("CAN.Device Number"=w126:u8)
          n63 = call <vilib>:"WPI_CANTalonSRX_SetParameter.vi"("Value"=0.0, "Parameter"=w127, "Device ID (0)"=w126) -> ()  [unwired: 7 in, 2 out]
        }
      }
    }
    frame "SHOOT" {
      n64 = call <vilib>:"WPI_CANTalonSRX_SetReference.vi"("error in (no error)"=w160, "Feedback Reference"=WPI_CANTalonSRX_APIFeedbackSelect."CTR Magnetic Enc (Relative)", "CAN Talon SRX Ref"=w161) -> ("error out"=w159:errorcluster, "CAN Talon SRX Ref"=w169:T4)  [unwired: 7 in]
      n65 = call <vilib>:"WPI_MotorControlSetOutput.vi"("error in (no error)"=w145, "Output"=0.75, "MotorControlDevRef"=w146) -> ("error out"=w142:errorcluster, "MotorControlDevRef"=w140:T4)  [unwired: 6 in, 1 out]
      n66 = call <vilib>:"WPI_CANTalonSRX_SetPID.vi"("CAN Talon SRX Ref"=w169, "P"=0.0, "I"=0.0, "D"=0.0, "error in (no error)"=w159, "F"=0.01, "I Zone"=0.0, "Ramp Rate"=0.0) -> ("CAN Talon SRX Ref"=w166:T4, "error out"=w158:errorcluster)  [unwired: 6 in]
      n67 = call <vilib>:"WPI_CANTalonSRX_ChangeMode.vi"("error in (no error)"=w158, "Output"=9800.0 ("y"), "Control Mode"=WPI_CANTalonSRX_APIControlMode."Speed", "CAN Talon SRX Ref"=w166) -> ("error out"=w157:errorcluster, "CAN Talon SRX Ref"=w162:T4)  [unwired: 6 in]
      n68 = call <vilib>:"WPI_CANTalonSRX_GetStatus.vi"("error in (no error)"=w157, "CAN Talon SRX Ref"=w162) -> ("error out"=w143:errorcluster)  [unwired: 7 in, 2 out]
      n69 = Merge Errors(w143, w142) -> (w141:errorcluster)
      n70 = call <vilib>:"WPI_RobotDriveDelayAndUpdateSafety.vi"("error in (no error)"=w141, "Delay (s)"=10.0, "RobotDriveDevRef"=w155) -> ("error out"=w139:errorcluster, "RobotDriveDevRef 2"=w156:T8)  [unwired: 7 in]
      n71 = call <vilib>:"WPI_MotorControlSetOutput.vi"("error in (no error)"=w139, "Output"=0.0, "MotorControlDevRef"=w140) -> ()  [unwired: 6 in, 3 out]
      n72 = call-poly <vilib>:"WPI_RobotDriveArcadeDrive.vi"("error in (no error)"=w139, "Y axis value"=0.0, "X axis value"=0.4, "RobotDriveDevRef"=w156) -> ("error out"=w152:errorcluster, "RobotDriveDevRef"=w153:T8)  [unwired: 5 in, 1 out]
      n73 = call <vilib>:"WPI_RobotDriveDelayAndUpdateSafety.vi"("error in (no error)"=w152, "Delay (s)"=1.0, "RobotDriveDevRef"=w153) -> ("error out"=w132:errorcluster, "RobotDriveDevRef 2"=w131:T8)  [unwired: 7 in]
      n74 = call-poly <vilib>:"WPI_RobotDriveArcadeDrive.vi"("error in (no error)"=w132, "Y axis value"=-0.6, "X axis value"=0.0, "RobotDriveDevRef"=w131) -> ("error out"=w135:errorcluster, "RobotDriveDevRef"=w136:T8)  [unwired: 5 in, 1 out]
      n75 = call <vilib>:"WPI_RobotDriveDelayAndUpdateSafety.vi"("error in (no error)"=w135, "Delay (s)"=3.0, "RobotDriveDevRef"=w136) -> ("error out"=w129:errorcluster, "RobotDriveDevRef 2"=w130:T8)  [unwired: 7 in]
      n76 = call-poly <vilib>:"WPI_RobotDriveArcadeDrive.vi"("error in (no error)"=w129, "Y axis value"=0.0, "X axis value"=0.0, "RobotDriveDevRef"=w130) -> ()  [unwired: 5 in, 3 out]
    }
    frame "SHOOTRED" {
      # "SHOOTRED"
      n77 = call <vilib>:"WPI_CANTalonSRX_SetReference.vi"("error in (no error)"=w226, "Feedback Reference"=WPI_CANTalonSRX_APIFeedbackSelect."CTR Magnetic Enc (Relative)", "CAN Talon SRX Ref"=w227) -> ("error out"=w225:errorcluster, "CAN Talon SRX Ref"=w235:T4)  [unwired: 7 in]
      n78 = call <vilib>:"WPI_MotorControlSetOutput.vi"("error in (no error)"=w213, "Output"=0.75, "MotorControlDevRef"=w214) -> ("error out"=w210:errorcluster, "MotorControlDevRef"=w208:T4)  [unwired: 6 in, 1 out]
      n79 = call <vilib>:"WPI_CANTalonSRX_SetPID.vi"("CAN Talon SRX Ref"=w235, "P"=0.0, "I"=0.0, "D"=0.0, "error in (no error)"=w225, "F"=0.01, "I Zone"=0.0, "Ramp Rate"=0.0) -> ("CAN Talon SRX Ref"=w232:T4, "error out"=w224:errorcluster)  [unwired: 6 in]
      n80 = call <vilib>:"WPI_CANTalonSRX_ChangeMode.vi"("error in (no error)"=w224, "Output"=9800.0 ("y"), "Control Mode"=WPI_CANTalonSRX_APIControlMode."Speed", "CAN Talon SRX Ref"=w232) -> ("error out"=w223:errorcluster, "CAN Talon SRX Ref"=w228:T4)  [unwired: 6 in]
      n81 = call <vilib>:"WPI_CANTalonSRX_GetStatus.vi"("error in (no error)"=w223, "CAN Talon SRX Ref"=w228) -> ("error out"=w211:errorcluster, "CAN Talon SRX Ref"=w193:T4)  [unwired: 7 in, 1 out]
      n82 = Merge Errors(w211, w210) -> (w209:errorcluster)
      n83 = call <vilib>:"WPI_RobotDriveDelayAndUpdateSafety.vi"("error in (no error)"=w209, "Delay (s)"=10.0, "RobotDriveDevRef"=w221) -> ("error out"=w192:errorcluster, "RobotDriveDevRef 2"=w222:T8)  [unwired: 7 in]
      n84 = call <vilib>:"WPI_CANTalonSRX_ChangeMode.vi"("error in (no error)"=w192, "Output"=0.0 ("y"), "Control Mode"=WPI_CANTalonSRX_APIControlMode."Speed", "CAN Talon SRX Ref"=w193) -> ("error out"=w194:errorcluster, "CAN Talon SRX Ref"=w195:T4)  [unwired: 6 in]
      n85 = call <vilib>:"WPI_MotorControlSetOutput.vi"("error in (no error)"=w192, "Output"=0.0, "MotorControlDevRef"=w208) -> ("error out"=w190:errorcluster)  [unwired: 6 in, 2 out]
      n86 = call <vilib>:"WPI_CANTalonSRX_GetStatus.vi"("error in (no error)"=w194, "CAN Talon SRX Ref"=w195) -> ("error out"=w191:errorcluster)  [unwired: 7 in, 2 out]
      n87 = Merge Errors(w191, w190) -> (w189:errorcluster)
      n88 = call <vilib>:"WPI_RobotDriveTankDrive.vi"("error in (no error)"=w189, "Right axis value"=0.6 ("Y axis value"), "Left axis value"=0.6, "RobotDriveDevRef"=w222) -> ("error out"=w219:errorcluster, "RobotDriveDevRef"=w220:T8)  [unwired: 5 in, 1 out]
      n89 = call <vilib>:"WPI_RobotDriveDelayAndUpdateSafety.vi"("error in (no error)"=w219, "Delay (s)"=0.25, "RobotDriveDevRef"=w220) -> ("error out"=w201:errorcluster, "RobotDriveDevRef 2"=w200:T8)  [unwired: 7 in]
      n90 = call-poly <vilib>:"WPI_RobotDriveArcadeDrive.vi"("error in (no error)"=w201, "Y axis value"=0.0, "X axis value"=-0.8, "RobotDriveDevRef"=w200) -> ("error out"=w204:errorcluster, "RobotDriveDevRef"=w205:T8)  [unwired: 5 in, 1 out]
      n91 = call <vilib>:"WPI_RobotDriveDelayAndUpdateSafety.vi"("error in (no error)"=w204, "Delay (s)"=0.5, "RobotDriveDevRef"=w205) -> ("error out"=w198:errorcluster, "RobotDriveDevRef 2"=w199:T8)  [unwired: 7 in]
      n92 = call-poly <vilib>:"WPI_RobotDriveArcadeDrive.vi"("error in (no error)"=w198, "Y axis value"=-0.5, "X axis value"=-0.55, "RobotDriveDevRef"=w199) -> ("error out"=w187:errorcluster, "RobotDriveDevRef"=w188:T8)  [unwired: 5 in, 1 out]
      n93 = call <vilib>:"WPI_RobotDriveDelayAndUpdateSafety.vi"("error in (no error)"=w187, "Delay (s)"=1.0, "RobotDriveDevRef"=w188) -> ("error out"=w185:errorcluster, "RobotDriveDevRef 2"=w184:T8)  [unwired: 7 in]
      n94 = call-poly <vilib>:"WPI_RobotDriveArcadeDrive.vi"("error in (no error)"=w185, "Y axis value"=-0.5 ("X axis value"), "RobotDriveDevRef"=w184) -> ("error out"=w179:errorcluster, "RobotDriveDevRef"=w180:T8)  [unwired: 6 in, 1 out]
      n95 = call <vilib>:"WPI_RobotDriveDelayAndUpdateSafety.vi"("error in (no error)"=w179, "Delay (s)"=2.0, "RobotDriveDevRef"=w180) -> ("error out"=w176:errorcluster, "RobotDriveDevRef 2"=w177:T8)  [unwired: 7 in]
      n96 = call-poly <vilib>:"WPI_RobotDriveArcadeDrive.vi"("error in (no error)"=w176, "Y axis value"=0.0, "X axis value"=0.0, "RobotDriveDevRef"=w177) -> ()  [unwired: 5 in, 3 out]
    }
    frame "MIDDLE" {
      n97 = call-poly <vilib>:"WPI_RobotDriveArcadeDrive.vi"("error in (no error)"=w269, "Y axis value"=0.45, "RobotDriveDevRef"=w270) -> ("error out"=w266:errorcluster, "RobotDriveDevRef"=w267:T8)  [unwired: 6 in, 1 out]
      n98 = call <vilib>:"WPI_RobotDriveDelayAndUpdateSafety.vi"("error in (no error)"=w266, "Delay (s)"=2.0, "RobotDriveDevRef"=w267) -> ("error out"=w264:errorcluster, "RobotDriveDevRef 2"=w263:T8)  [unwired: 7 in]
      n99 = call-poly <vilib>:"WPI_RobotDriveArcadeDrive.vi"("error in (no error)"=w264, "Y axis value"=0.0, "RobotDriveDevRef"=w263) -> ("error out"=w260:errorcluster, "RobotDriveDevRef"=w261:T8)  [unwired: 6 in, 1 out]
      n100 = call <vilib>:"WPI_RobotDriveDelayAndUpdateSafety.vi"("error in (no error)"=w260, "Delay (s)"=0.5, "RobotDriveDevRef"=w261) -> ("error out"=w258:errorcluster, "RobotDriveDevRef 2"=w256:T8)  [unwired: 7 in]
      n101 = call <vilib>:"WPI_MotorControlSetOutput.vi"("error in (no error)"=w258, "Output"=-0.7, "MotorControlDevRef"=w257) -> ("error out"=w255:errorcluster, "MotorControlDevRef"=w251:T4)  [unwired: 6 in, 1 out]
      n102 = call <vilib>:"WPI_RobotDriveDelayAndUpdateSafety.vi"("error in (no error)"=w255, "Delay (s)"=1.5, "RobotDriveDevRef"=w256) -> ("error out"=w252:errorcluster, "RobotDriveDevRef 2"=w249:T8)  [unwired: 7 in]
      n103 = call <vilib>:"WPI_MotorControlSetOutput.vi"("error in (no error)"=w252, "Output"=0.0, "MotorControlDevRef"=w251) -> ("error out"=w248:errorcluster)  [unwired: 6 in, 2 out]
      n104 = call-poly <vilib>:"WPI_RobotDriveArcadeDrive.vi"("error in (no error)"=w248, "Y axis value"=-0.4, "RobotDriveDevRef"=w249) -> ("error out"=w245:errorcluster, "RobotDriveDevRef"=w246:T8)  [unwired: 6 in, 1 out]
      n105 = call <vilib>:"WPI_RobotDriveDelayAndUpdateSafety.vi"("error in (no error)"=w245, "Delay (s)"=2.0, "RobotDriveDevRef"=w246) -> ("error out"=w242:errorcluster, "RobotDriveDevRef 2"=w243:T8)  [unwired: 7 in]
      n106 = call-poly <vilib>:"WPI_RobotDriveArcadeDrive.vi"("error in (no error)"=w242, "Y axis value"=0.0, "X axis value"=0.0, "RobotDriveDevRef"=w243) -> ()  [unwired: 5 in, 3 out]
    }
    frame "RIGHTSIDE" {
      # "RIGHTSIDE"
      n107 = call-poly <vilib>:"WPI_RobotDriveArcadeDrive.vi"("error in (no error)"=w272, "Y axis value"=0.59, "RobotDriveDevRef"=w273) -> ("error out"=w312:errorcluster, "RobotDriveDevRef"=w313:T8)  [unwired: 6 in, 1 out]
      n108 = call <vilib>:"WPI_RobotDriveDelayAndUpdateSafety.vi"("error in (no error)"=w312, "Delay (s)"=1.8, "RobotDriveDevRef"=w313) -> ("error out"=w308:errorcluster, "RobotDriveDevRef 2"=w309:T8)  [unwired: 7 in]
      n109 = call-poly <vilib>:"WPI_RobotDriveArcadeDrive.vi"("error in (no error)"=w308, "X axis value"=0.36, "RobotDriveDevRef"=w309) -> ("error out"=w305:errorcluster, "RobotDriveDevRef"=w306:T8)  [unwired: 6 in, 1 out]
      n110 = call <vilib>:"WPI_RobotDriveDelayAndUpdateSafety.vi"("error in (no error)"=w305, "Delay (s)"=1.0, "RobotDriveDevRef"=w306) -> ("error out"=w302:errorcluster, "RobotDriveDevRef 2"=w303:T8)  [unwired: 7 in]
      n111 = call-poly <vilib>:"WPI_RobotDriveArcadeDrive.vi"("error in (no error)"=w302, "Y axis value"=0.5, "RobotDriveDevRef"=w303) -> ("error out"=w299:errorcluster, "RobotDriveDevRef"=w300:T8)  [unwired: 6 in, 1 out]
      n112 = call <vilib>:"WPI_RobotDriveDelayAndUpdateSafety.vi"("error in (no error)"=w299, "Delay (s)"=2.3, "RobotDriveDevRef"=w300) -> ("error out"=w296:errorcluster, "RobotDriveDevRef 2"=w297:T8)  [unwired: 7 in]
      n113 = call-poly <vilib>:"WPI_RobotDriveArcadeDrive.vi"("error in (no error)"=w296, "Y axis value"=0.0, "RobotDriveDevRef"=w297) -> ("error out"=w293:errorcluster, "RobotDriveDevRef"=w294:T8)  [unwired: 6 in, 1 out]
      n114 = call <vilib>:"WPI_RobotDriveDelayAndUpdateSafety.vi"("error in (no error)"=w293, "Delay (s)"=0.5, "RobotDriveDevRef"=w294) -> ("error out"=w291:errorcluster, "RobotDriveDevRef 2"=w289:T8)  [unwired: 7 in]
      n115 = call <vilib>:"WPI_MotorControlSetOutput.vi"("error in (no error)"=w291, "Output"=-0.7, "MotorControlDevRef"=w271) -> ("error out"=w288:errorcluster, "MotorControlDevRef"=w277:T4)  [unwired: 6 in, 1 out]
      n116 = call <vilib>:"WPI_RobotDriveDelayAndUpdateSafety.vi"("error in (no error)"=w288, "Delay (s)"=1.5, "RobotDriveDevRef"=w289) -> ("error out"=w276:errorcluster, "RobotDriveDevRef 2"=w286:T8)  [unwired: 7 in]
      n117 = call <vilib>:"WPI_MotorControlSetOutput.vi"("error in (no error)"=w276, "Output"=0.0, "MotorControlDevRef"=w277) -> ("error out"=w274:errorcluster)  [unwired: 6 in, 2 out]
      n118 = call-poly <vilib>:"WPI_RobotDriveArcadeDrive.vi"("error in (no error)"=w274, "Y axis value"=-0.4, "RobotDriveDevRef"=w286) -> ("error out"=w283:errorcluster, "RobotDriveDevRef"=w284:T8)  [unwired: 6 in, 1 out]
      n119 = call <vilib>:"WPI_RobotDriveDelayAndUpdateSafety.vi"("error in (no error)"=w283, "Delay (s)"=2.0, "RobotDriveDevRef"=w284) -> ("error out"=w281:errorcluster, "RobotDriveDevRef 2"=w280:T8)  [unwired: 7 in]
      n120 = call-poly <vilib>:"WPI_RobotDriveArcadeDrive.vi"("error in (no error)"=w281, "Y axis value"=0.0, "X axis value"=0.0, "RobotDriveDevRef"=w280) -> ()  [unwired: 5 in, 3 out]
    }
    frame "LEFTSIDE" {
      n121 = call-poly <vilib>:"WPI_RobotDriveArcadeDrive.vi"("error in (no error)"=w355, "Y axis value"=0.6, "RobotDriveDevRef"=w356) -> ("error out"=w353:errorcluster, "RobotDriveDevRef"=w354:T8)  [unwired: 6 in, 1 out]
      n122 = call <vilib>:"WPI_RobotDriveDelayAndUpdateSafety.vi"("error in (no error)"=w353, "Delay (s)"=2.0, "RobotDriveDevRef"=w354) -> ("error out"=w349:errorcluster, "RobotDriveDevRef 2"=w350:T8)  [unwired: 7 in]
      n123 = call-poly <vilib>:"WPI_RobotDriveArcadeDrive.vi"("error in (no error)"=w349, "X axis value"=-0.45, "RobotDriveDevRef"=w350) -> ("error out"=w346:errorcluster, "RobotDriveDevRef"=w347:T8)  [unwired: 6 in, 1 out]
      n124 = call <vilib>:"WPI_RobotDriveDelayAndUpdateSafety.vi"("error in (no error)"=w346, "Delay (s)"=1.0, "RobotDriveDevRef"=w347) -> ("error out"=w343:errorcluster, "RobotDriveDevRef 2"=w344:T8)  [unwired: 7 in]
      n125 = call-poly <vilib>:"WPI_RobotDriveArcadeDrive.vi"("error in (no error)"=w343, "Y axis value"=0.52, "RobotDriveDevRef"=w344) -> ("error out"=w340:errorcluster, "RobotDriveDevRef"=w341:T8)  [unwired: 6 in, 1 out]
      n126 = call <vilib>:"WPI_RobotDriveDelayAndUpdateSafety.vi"("error in (no error)"=w340, "Delay (s)"=2.25, "RobotDriveDevRef"=w341) -> ("error out"=w337:errorcluster, "RobotDriveDevRef 2"=w338:T8)  [unwired: 7 in]
      n127 = call-poly <vilib>:"WPI_RobotDriveArcadeDrive.vi"("error in (no error)"=w337, "Y axis value"=0.0, "RobotDriveDevRef"=w338) -> ("error out"=w334:errorcluster, "RobotDriveDevRef"=w335:T8)  [unwired: 6 in, 1 out]
      n128 = call <vilib>:"WPI_RobotDriveDelayAndUpdateSafety.vi"("error in (no error)"=w334, "Delay (s)"=0.5, "RobotDriveDevRef"=w335) -> ("error out"=w331:errorcluster, "RobotDriveDevRef 2"=w329:T8)  [unwired: 7 in]
      n129 = call <vilib>:"WPI_MotorControlSetOutput.vi"("error in (no error)"=w331, "Output"=-0.7, "MotorControlDevRef"=w332) -> ("error out"=w328:errorcluster, "MotorControlDevRef"=w317:T4)  [unwired: 6 in, 1 out]
      n130 = call <vilib>:"WPI_RobotDriveDelayAndUpdateSafety.vi"("error in (no error)"=w328, "Delay (s)"=1.5, "RobotDriveDevRef"=w329) -> ("error out"=w316:errorcluster, "RobotDriveDevRef 2"=w326:T8)  [unwired: 7 in]
      n131 = call <vilib>:"WPI_MotorControlSetOutput.vi"("error in (no error)"=w316, "Output"=0.0, "MotorControlDevRef"=w317) -> ("error out"=w314:errorcluster)  [unwired: 6 in, 2 out]
      n132 = call-poly <vilib>:"WPI_RobotDriveArcadeDrive.vi"("error in (no error)"=w314, "Y axis value"=-0.4, "RobotDriveDevRef"=w326) -> ("error out"=w323:errorcluster, "RobotDriveDevRef"=w324:T8)  [unwired: 6 in, 1 out]
      n133 = call <vilib>:"WPI_RobotDriveDelayAndUpdateSafety.vi"("error in (no error)"=w323, "Delay (s)"=2.0, "RobotDriveDevRef"=w324) -> ("error out"=w321:errorcluster, "RobotDriveDevRef 2"=w320:T8)  [unwired: 7 in]
      n134 = call-poly <vilib>:"WPI_RobotDriveArcadeDrive.vi"("error in (no error)"=w321, "Y axis value"=0.0, "X axis value"=0.0, "RobotDriveDevRef"=w320) -> ()  [unwired: 5 in, 3 out]
    }
    frame "A" {
      n135 = flat-sequence {
        tunnel: w361 -> [w376]
        tunnel: w362 -> [w377]
        tunnel: [w377] -> w374
        tunnel: [w376] -> w373
        tunnel: w374 -> [w386]
        tunnel: w373 -> [w385]
        tunnel: [w384] -> w372
        tunnel: [w383] -> w371
        tunnel: w372 -> [w409]
        tunnel: w371 -> [w408]
        tunnel: [w409] -> w370
        tunnel: [w408] -> w369
        tunnel: [w417] -> w358
        tunnel: [w416] -> w357
        tunnel: w369 -> [w418]
        tunnel: w370 -> [w419]
        tunnel: [w442] -> w368
        tunnel: [w441] -> w367
        tunnel: w357 -> [w441]
        tunnel: w358 -> [w442]
        tunnel: w368 -> [w450]
        tunnel: w367 -> [w451]
        tunnel: [w450] -> w366
        tunnel: [w449] -> w364
        tunnel: w366 -> [w462]
        tunnel: [w462] -> w365
        tunnel: w364 -> [w466]
        tunnel: [w466] -> w363
        tunnel: w365 -> [w472]
        tunnel: w363 -> [w473]
        tunnel: [w471] -> w359
        tunnel: [w470] -> w360
        tunnel: w359 -> [w496]
        tunnel: w360 -> [w498]
        frame #0 {
          w378 = T10 77 items=["Slot 0 - P"=1, "Slot 0 - I"=2, "Slot 0 - D"=3, "Slot 0 - F"=4, "Slot 0 - I Zone"=5, "Slot 0 - Ramp Rate"=6, "Slot 1 - P"=11, "Slot 1 - I"=12, "Slot 1 - D"=13, "Slot 1 - F"=14, "Slot 1 - I Zone"=15, "Slot 1 - Ramp Rate"=16, "Soft Limit - Forward"=21, "Soft Limit - Reverse"=22, "Soft Limit - Forward Enable"=23, "Soft Limit - Reverse Enable"=24, "On Boot - Brake Mode"=31, "On Boot - Limit Normally Closed - Forward"=32, "On Boot - Limit Normally Closed - Reverse"=33, "On Boot - Limit Disabled - Forward"=34, "On Boot - Limit Disabled - Reverse"=35, "Fault - Over Temp"=41, "Fault - Under Voltage"=42, "Fault - Forward Limit"=43, "Fault - Reverse Limit"=44, "Fault - Hardware Failure"=45, "Fault - Forward Soft Limit"=46, "Fault - Reverse Soft Limit"=47, "Sticky Fault - Over Temp"=48, "Sticky Fault - Under Voltage"=49, "Sticky Fault - Forward Limit"=50, "Sticky Fault - Reverse Limit"=51, "Sticky Fault - Forward Soft Limit"=52, "Sticky Fault - Reverse Soft Limit"=53, "Applied Throttle"=61, "Closed-Loop Error"=62, "Select Feedback Device"=63, "Reverse Closed-Loop Output"=64, "Mode Select"=65, "Profile Slot Select"=66, "Ramp Throttle"=67, "Reverse Feedback Sensor"=68, "Limit Switch Enabled"=69, "Limit Switch Closed - Forward"=70, "Limit Switch Closed - Reverse"=71, "Sensor Position"=73, "Sensor Velocity"=74, "Current"=75, "Brake is Enabled"=76, "Encoder Position"=77, "Encoder Velocity"=78, "Encoder Index Rise Events"=79, "Encoder A Pin State"=80, "Encoder B Pin State"=81, "Encoder Index Pin State"=82, "Analog In with Overflow"=83, "Analog In Velocity"=84, "Temperature"=85, "Battery Voltage"=86, "Reset Count"=87, "Reset Flags"=88, "Firmware Version"=89, "Settings Changed"=90, "Quad Filter Enable"=91, "Ignore Disable Broadcast"=92, "I Accumulator"=93, "Status 1 Frame Rate Ms"=94, "Status 2 Frame Rate Ms"=95, "Status 3 Frame Rate Ms"=96, "Status 4 Frame Rate Ms"=97, "Status 6 Frame Rate Ms"=98, "Status 7 Frame Rate Ms"=99, "Enable Index Pin Clear Position"=100, "Peak Positive Output"=104, "Nominal Positive Output"=105, "Peak Negative Output"=106, "Nominal Negative Output"=107, "Quad Index Pin Polarity"=108, "Status 8 Frame Rate Ms"=109, "Allow Position Overflow"=110, "Slot 0 - Allowable Closed-Loop Error"=111, "Number Potentiometer Turns"=112, "Encoder Codes Per Rev"=113, "Pulse Width Decoded Position"=114, "Analog Position"=115, "Voltage Compensation Rate (V/s)"=116, "Slot 1 - Allowable Closed-Loop Error"=117, "Motion Profile Has Underrun Err"=119, "Reserved 120"=120, "Legacy Control Mode"=121, "Motion Magic Acceleration"=122, "Motion Magic Cruise Velocity"=123, "Status 10 Frame Rate"=124, "Current Limit Threshold"=125, "CustomParam0"=137, "CustomParam1"=138, "PersStorageSaving"=139, "ClearPositionOnLimitF"=144, "ClearPositionOnLimitR"=145, "NominalBatteryVoltage"=146, "SampleVelocityPeriod"=147, "SampleVelocityWindow"=148] ("Parameter")
          w381 = T10 77 items=["Slot 0 - P"=1, "Slot 0 - I"=2, "Slot 0 - D"=3, "Slot 0 - F"=4, "Slot 0 - I Zone"=5, "Slot 0 - Ramp Rate"=6, "Slot 1 - P"=11, "Slot 1 - I"=12, "Slot 1 - D"=13, "Slot 1 - F"=14, "Slot 1 - I Zone"=15, "Slot 1 - Ramp Rate"=16, "Soft Limit - Forward"=21, "Soft Limit - Reverse"=22, "Soft Limit - Forward Enable"=23, "Soft Limit - Reverse Enable"=24, "On Boot - Brake Mode"=31, "On Boot - Limit Normally Closed - Forward"=32, "On Boot - Limit Normally Closed - Reverse"=33, "On Boot - Limit Disabled - Forward"=34, "On Boot - Limit Disabled - Reverse"=35, "Fault - Over Temp"=41, "Fault - Under Voltage"=42, "Fault - Forward Limit"=43, "Fault - Reverse Limit"=44, "Fault - Hardware Failure"=45, "Fault - Forward Soft Limit"=46, "Fault - Reverse Soft Limit"=47, "Sticky Fault - Over Temp"=48, "Sticky Fault - Under Voltage"=49, "Sticky Fault - Forward Limit"=50, "Sticky Fault - Reverse Limit"=51, "Sticky Fault - Forward Soft Limit"=52, "Sticky Fault - Reverse Soft Limit"=53, "Applied Throttle"=61, "Closed-Loop Error"=62, "Select Feedback Device"=63, "Reverse Closed-Loop Output"=64, "Mode Select"=65, "Profile Slot Select"=66, "Ramp Throttle"=67, "Reverse Feedback Sensor"=68, "Limit Switch Enabled"=69, "Limit Switch Closed - Forward"=70, "Limit Switch Closed - Reverse"=71, "Sensor Position"=73, "Sensor Velocity"=74, "Current"=75, "Brake is Enabled"=76, "Encoder Position"=77, "Encoder Velocity"=78, "Encoder Index Rise Events"=79, "Encoder A Pin State"=80, "Encoder B Pin State"=81, "Encoder Index Pin State"=82, "Analog In with Overflow"=83, "Analog In Velocity"=84, "Temperature"=85, "Battery Voltage"=86, "Reset Count"=87, "Reset Flags"=88, "Firmware Version"=89, "Settings Changed"=90, "Quad Filter Enable"=91, "Ignore Disable Broadcast"=92, "I Accumulator"=93, "Status 1 Frame Rate Ms"=94, "Status 2 Frame Rate Ms"=95, "Status 3 Frame Rate Ms"=96, "Status 4 Frame Rate Ms"=97, "Status 6 Frame Rate Ms"=98, "Status 7 Frame Rate Ms"=99, "Enable Index Pin Clear Position"=100, "Peak Positive Output"=104, "Nominal Positive Output"=105, "Peak Negative Output"=106, "Nominal Negative Output"=107, "Quad Index Pin Polarity"=108, "Status 8 Frame Rate Ms"=109, "Allow Position Overflow"=110, "Slot 0 - Allowable Closed-Loop Error"=111, "Number Potentiometer Turns"=112, "Encoder Codes Per Rev"=113, "Pulse Width Decoded Position"=114, "Analog Position"=115, "Voltage Compensation Rate (V/s)"=116, "Slot 1 - Allowable Closed-Loop Error"=117, "Motion Profile Has Underrun Err"=119, "Reserved 120"=120, "Legacy Control Mode"=121, "Motion Magic Acceleration"=122, "Motion Magic Cruise Velocity"=123, "Status 10 Frame Rate"=124, "Current Limit Threshold"=125, "CustomParam0"=137, "CustomParam1"=138, "PersStorageSaving"=139, "ClearPositionOnLimitF"=144, "ClearPositionOnLimitR"=145, "NominalBatteryVoltage"=146, "SampleVelocityPeriod"=147, "SampleVelocityWindow"=148] ("Parameter")
          n136 = Unbundle By Name(w376) -> ("CAN.Device Number"=w375:u8)
          n137 = Unbundle By Name(w377) -> ("CAN.Device Number"=w382:u8)
          n138 = call <vilib>:"WPI_CANTalonSRX_SetParameter.vi"("Value"=0.0, "Parameter"=w378, "Device ID (0)"=w375) -> ()  [unwired: 7 in, 2 out]
          n139 = call <vilib>:"WPI_CANTalonSRX_SetParameter.vi"("Value"=0.0, "Parameter"=w381, "Device ID (0)"=w382) -> ()  [unwired: 7 in, 2 out]
        }
        frame #1 {
          n140 = while {
            tunnel: w386 -> [w392]
            tunnel: w385 -> [w399]
            tunnel: [w398] -> w383
            tunnel: [w397] -> w384
            stop <- w389 stop-if-true
            n141 = call <vilib>:"WPI_CANTalonSRX_GetStatus.vi"("CAN Talon SRX Ref"=w392) -> ("Talon SRX Status"=w395:T11, "CAN Talon SRX Ref"=w390:T4)  [unwired: 8 in, 1 out]
            n142 = call <vilib>:"WPI_CANTalonSRX_GetStatus.vi"("CAN Talon SRX Ref"=w399) -> ("Talon SRX Status"=w400:T11, "CAN Talon SRX Ref"=w401:T4)  [unwired: 8 in, 1 out]
            n143 = Unbundle By Name(w395) -> ("Encoder Position"=w394:dbl)
            "Encoder Position 7" <- w394
            n144 = Unbundle By Name(w400) -> ("Encoder Position"=w402:dbl)
            "Encoder Position 6" <- w402
            n145 = Less?(x=-2256.0, y=w394) -> (x < y?=w387:bool)
            n146 = Greater?(x=5325.0, y=w402) -> (0:w388:bool)
            n147 = And(x=w387, y=w388) -> (x .and. y?=w389:bool)
            n148 = case shown="True" w387 {
              tunnel: [0.0 ("Output") 0.2 ("Output")] -> w391
              frame False {
              }
              frame True {
              }
            }
            n149 = case shown="True" w388 {
              tunnel: [0.0 ("Output") 0.2 ("Output")] -> w396
              frame False {
              }
              frame True {
              }
            }
            n150 = call <vilib>:"WPI_MotorControlSetOutput.vi"("Output"=w391, "MotorControlDevRef"=w390) -> ("MotorControlDevRef"=w397:T4)  [unwired: 7 in, 2 out]
            n151 = call <vilib>:"WPI_MotorControlSetOutput.vi"("Output"=w396, "MotorControlDevRef"=w401) -> ("MotorControlDevRef"=w398:T4)  [unwired: 7 in, 2 out]
          }
        }
        frame #2 {
          w414 = T10 77 items=["Slot 0 - P"=1, "Slot 0 - I"=2, "Slot 0 - D"=3, "Slot 0 - F"=4, "Slot 0 - I Zone"=5, "Slot 0 - Ramp Rate"=6, "Slot 1 - P"=11, "Slot 1 - I"=12, "Slot 1 - D"=13, "Slot 1 - F"=14, "Slot 1 - I Zone"=15, "Slot 1 - Ramp Rate"=16, "Soft Limit - Forward"=21, "Soft Limit - Reverse"=22, "Soft Limit - Forward Enable"=23, "Soft Limit - Reverse Enable"=24, "On Boot - Brake Mode"=31, "On Boot - Limit Normally Closed - Forward"=32, "On Boot - Limit Normally Closed - Reverse"=33, "On Boot - Limit Disabled - Forward"=34, "On Boot - Limit Disabled - Reverse"=35, "Fault - Over Temp"=41, "Fault - Under Voltage"=42, "Fault - Forward Limit"=43, "Fault - Reverse Limit"=44, "Fault - Hardware Failure"=45, "Fault - Forward Soft Limit"=46, "Fault - Reverse Soft Limit"=47, "Sticky Fault - Over Temp"=48, "Sticky Fault - Under Voltage"=49, "Sticky Fault - Forward Limit"=50, "Sticky Fault - Reverse Limit"=51, "Sticky Fault - Forward Soft Limit"=52, "Sticky Fault - Reverse Soft Limit"=53, "Applied Throttle"=61, "Closed-Loop Error"=62, "Select Feedback Device"=63, "Reverse Closed-Loop Output"=64, "Mode Select"=65, "Profile Slot Select"=66, "Ramp Throttle"=67, "Reverse Feedback Sensor"=68, "Limit Switch Enabled"=69, "Limit Switch Closed - Forward"=70, "Limit Switch Closed - Reverse"=71, "Sensor Position"=73, "Sensor Velocity"=74, "Current"=75, "Brake is Enabled"=76, "Encoder Position"=77, "Encoder Velocity"=78, "Encoder Index Rise Events"=79, "Encoder A Pin State"=80, "Encoder B Pin State"=81, "Encoder Index Pin State"=82, "Analog In with Overflow"=83, "Analog In Velocity"=84, "Temperature"=85, "Battery Voltage"=86, "Reset Count"=87, "Reset Flags"=88, "Firmware Version"=89, "Settings Changed"=90, "Quad Filter Enable"=91, "Ignore Disable Broadcast"=92, "I Accumulator"=93, "Status 1 Frame Rate Ms"=94, "Status 2 Frame Rate Ms"=95, "Status 3 Frame Rate Ms"=96, "Status 4 Frame Rate Ms"=97, "Status 6 Frame Rate Ms"=98, "Status 7 Frame Rate Ms"=99, "Enable Index Pin Clear Position"=100, "Peak Positive Output"=104, "Nominal Positive Output"=105, "Peak Negative Output"=106, "Nominal Negative Output"=107, "Quad Index Pin Polarity"=108, "Status 8 Frame Rate Ms"=109, "Allow Position Overflow"=110, "Slot 0 - Allowable Closed-Loop Error"=111, "Number Potentiometer Turns"=112, "Encoder Codes Per Rev"=113, "Pulse Width Decoded Position"=114, "Analog Position"=115, "Voltage Compensation Rate (V/s)"=116, "Slot 1 - Allowable Closed-Loop Error"=117, "Motion Profile Has Underrun Err"=119, "Reserved 120"=120, "Legacy Control Mode"=121, "Motion Magic Acceleration"=122, "Motion Magic Cruise Velocity"=123, "Status 10 Frame Rate"=124, "Current Limit Threshold"=125, "CustomParam0"=137, "CustomParam1"=138, "PersStorageSaving"=139, "ClearPositionOnLimitF"=144, "ClearPositionOnLimitR"=145, "NominalBatteryVoltage"=146, "SampleVelocityPeriod"=147, "SampleVelocityWindow"=148] ("Parameter")
          w411 = T10 77 items=["Slot 0 - P"=1, "Slot 0 - I"=2, "Slot 0 - D"=3, "Slot 0 - F"=4, "Slot 0 - I Zone"=5, "Slot 0 - Ramp Rate"=6, "Slot 1 - P"=11, "Slot 1 - I"=12, "Slot 1 - D"=13, "Slot 1 - F"=14, "Slot 1 - I Zone"=15, "Slot 1 - Ramp Rate"=16, "Soft Limit - Forward"=21, "Soft Limit - Reverse"=22, "Soft Limit - Forward Enable"=23, "Soft Limit - Reverse Enable"=24, "On Boot - Brake Mode"=31, "On Boot - Limit Normally Closed - Forward"=32, "On Boot - Limit Normally Closed - Reverse"=33, "On Boot - Limit Disabled - Forward"=34, "On Boot - Limit Disabled - Reverse"=35, "Fault - Over Temp"=41, "Fault - Under Voltage"=42, "Fault - Forward Limit"=43, "Fault - Reverse Limit"=44, "Fault - Hardware Failure"=45, "Fault - Forward Soft Limit"=46, "Fault - Reverse Soft Limit"=47, "Sticky Fault - Over Temp"=48, "Sticky Fault - Under Voltage"=49, "Sticky Fault - Forward Limit"=50, "Sticky Fault - Reverse Limit"=51, "Sticky Fault - Forward Soft Limit"=52, "Sticky Fault - Reverse Soft Limit"=53, "Applied Throttle"=61, "Closed-Loop Error"=62, "Select Feedback Device"=63, "Reverse Closed-Loop Output"=64, "Mode Select"=65, "Profile Slot Select"=66, "Ramp Throttle"=67, "Reverse Feedback Sensor"=68, "Limit Switch Enabled"=69, "Limit Switch Closed - Forward"=70, "Limit Switch Closed - Reverse"=71, "Sensor Position"=73, "Sensor Velocity"=74, "Current"=75, "Brake is Enabled"=76, "Encoder Position"=77, "Encoder Velocity"=78, "Encoder Index Rise Events"=79, "Encoder A Pin State"=80, "Encoder B Pin State"=81, "Encoder Index Pin State"=82, "Analog In with Overflow"=83, "Analog In Velocity"=84, "Temperature"=85, "Battery Voltage"=86, "Reset Count"=87, "Reset Flags"=88, "Firmware Version"=89, "Settings Changed"=90, "Quad Filter Enable"=91, "Ignore Disable Broadcast"=92, "I Accumulator"=93, "Status 1 Frame Rate Ms"=94, "Status 2 Frame Rate Ms"=95, "Status 3 Frame Rate Ms"=96, "Status 4 Frame Rate Ms"=97, "Status 6 Frame Rate Ms"=98, "Status 7 Frame Rate Ms"=99, "Enable Index Pin Clear Position"=100, "Peak Positive Output"=104, "Nominal Positive Output"=105, "Peak Negative Output"=106, "Nominal Negative Output"=107, "Quad Index Pin Polarity"=108, "Status 8 Frame Rate Ms"=109, "Allow Position Overflow"=110, "Slot 0 - Allowable Closed-Loop Error"=111, "Number Potentiometer Turns"=112, "Encoder Codes Per Rev"=113, "Pulse Width Decoded Position"=114, "Analog Position"=115, "Voltage Compensation Rate (V/s)"=116, "Slot 1 - Allowable Closed-Loop Error"=117, "Motion Profile Has Underrun Err"=119, "Reserved 120"=120, "Legacy Control Mode"=121, "Motion Magic Acceleration"=122, "Motion Magic Cruise Velocity"=123, "Status 10 Frame Rate"=124, "Current Limit Threshold"=125, "CustomParam0"=137, "CustomParam1"=138, "PersStorageSaving"=139, "ClearPositionOnLimitF"=144, "ClearPositionOnLimitR"=145, "NominalBatteryVoltage"=146, "SampleVelocityPeriod"=147, "SampleVelocityWindow"=148] ("Parameter")
          n152 = Unbundle By Name(w408) -> ("CAN.Device Number"=w415:u8)
          n153 = Unbundle By Name(w409) -> ("CAN.Device Number"=w410:u8)
          n154 = call <vilib>:"WPI_CANTalonSRX_SetParameter.vi"("Value"=0.0, "Parameter"=w414, "Device ID (0)"=w415) -> ()  [unwired: 7 in, 2 out]
          n155 = call <vilib>:"WPI_CANTalonSRX_SetParameter.vi"("Value"=0.0, "Parameter"=w411, "Device ID (0)"=w410) -> ()  [unwired: 7 in, 2 out]
        }
        frame #3 {
          n156 = while {
            tunnel: w419 -> [w436]
            tunnel: w418 -> [w425]
            tunnel: [w421] -> w417
            tunnel: [w420] -> w416
            stop <- w422 stop-if-true
            n157 = call <vilib>:"WPI_CANTalonSRX_GetStatus.vi"("CAN Talon SRX Ref"=w436) -> ("Talon SRX Status"=w435:T11, "CAN Talon SRX Ref"=w434:T4)  [unwired: 8 in, 1 out]
            n158 = call <vilib>:"WPI_CANTalonSRX_GetStatus.vi"("CAN Talon SRX Ref"=w425) -> ("Talon SRX Status"=w426:T11, "CAN Talon SRX Ref"=w427:T4)  [unwired: 8 in, 1 out]
            n159 = Unbundle By Name(w435) -> ("Encoder Position"=w433:dbl)
            n160 = Unbundle By Name(w426) -> ("Encoder Position"=w428:dbl)
            n161 = Greater?(x=1980.0, y=w433) -> (0:w423:bool)
            n162 = Less?(x=-4125.0, y=w428) -> (x < y?=w424:bool)
            n163 = case shown="False" w423 {
              tunnel: [-0.3 ("Output") 0.0 ("Output")] -> w431
              frame False {
              }
              frame True {
              }
            }
            n164 = case shown="False" w424 {
              tunnel: [-0.3 ("Output") 0.0 ("Output")] -> w430
              frame False {
              }
              frame True {
              }
            }
            n165 = And(x=w423, y=w424) -> (x .and. y?=w422:bool)
            n166 = call <vilib>:"WPI_MotorControlSetOutput.vi"("Output"=w431, "MotorControlDevRef"=w434) -> ("MotorControlDevRef"=w420:T4)  [unwired: 7 in, 2 out]
            n167 = call <vilib>:"WPI_MotorControlSetOutput.vi"("Output"=w430, "MotorControlDevRef"=w427) -> ("MotorControlDevRef"=w421:T4)  [unwired: 7 in, 2 out]
          }
        }
        frame #4 {
          w447 = T10 77 items=["Slot 0 - P"=1, "Slot 0 - I"=2, "Slot 0 - D"=3, "Slot 0 - F"=4, "Slot 0 - I Zone"=5, "Slot 0 - Ramp Rate"=6, "Slot 1 - P"=11, "Slot 1 - I"=12, "Slot 1 - D"=13, "Slot 1 - F"=14, "Slot 1 - I Zone"=15, "Slot 1 - Ramp Rate"=16, "Soft Limit - Forward"=21, "Soft Limit - Reverse"=22, "Soft Limit - Forward Enable"=23, "Soft Limit - Reverse Enable"=24, "On Boot - Brake Mode"=31, "On Boot - Limit Normally Closed - Forward"=32, "On Boot - Limit Normally Closed - Reverse"=33, "On Boot - Limit Disabled - Forward"=34, "On Boot - Limit Disabled - Reverse"=35, "Fault - Over Temp"=41, "Fault - Under Voltage"=42, "Fault - Forward Limit"=43, "Fault - Reverse Limit"=44, "Fault - Hardware Failure"=45, "Fault - Forward Soft Limit"=46, "Fault - Reverse Soft Limit"=47, "Sticky Fault - Over Temp"=48, "Sticky Fault - Under Voltage"=49, "Sticky Fault - Forward Limit"=50, "Sticky Fault - Reverse Limit"=51, "Sticky Fault - Forward Soft Limit"=52, "Sticky Fault - Reverse Soft Limit"=53, "Applied Throttle"=61, "Closed-Loop Error"=62, "Select Feedback Device"=63, "Reverse Closed-Loop Output"=64, "Mode Select"=65, "Profile Slot Select"=66, "Ramp Throttle"=67, "Reverse Feedback Sensor"=68, "Limit Switch Enabled"=69, "Limit Switch Closed - Forward"=70, "Limit Switch Closed - Reverse"=71, "Sensor Position"=73, "Sensor Velocity"=74, "Current"=75, "Brake is Enabled"=76, "Encoder Position"=77, "Encoder Velocity"=78, "Encoder Index Rise Events"=79, "Encoder A Pin State"=80, "Encoder B Pin State"=81, "Encoder Index Pin State"=82, "Analog In with Overflow"=83, "Analog In Velocity"=84, "Temperature"=85, "Battery Voltage"=86, "Reset Count"=87, "Reset Flags"=88, "Firmware Version"=89, "Settings Changed"=90, "Quad Filter Enable"=91, "Ignore Disable Broadcast"=92, "I Accumulator"=93, "Status 1 Frame Rate Ms"=94, "Status 2 Frame Rate Ms"=95, "Status 3 Frame Rate Ms"=96, "Status 4 Frame Rate Ms"=97, "Status 6 Frame Rate Ms"=98, "Status 7 Frame Rate Ms"=99, "Enable Index Pin Clear Position"=100, "Peak Positive Output"=104, "Nominal Positive Output"=105, "Peak Negative Output"=106, "Nominal Negative Output"=107, "Quad Index Pin Polarity"=108, "Status 8 Frame Rate Ms"=109, "Allow Position Overflow"=110, "Slot 0 - Allowable Closed-Loop Error"=111, "Number Potentiometer Turns"=112, "Encoder Codes Per Rev"=113, "Pulse Width Decoded Position"=114, "Analog Position"=115, "Voltage Compensation Rate (V/s)"=116, "Slot 1 - Allowable Closed-Loop Error"=117, "Motion Profile Has Underrun Err"=119, "Reserved 120"=120, "Legacy Control Mode"=121, "Motion Magic Acceleration"=122, "Motion Magic Cruise Velocity"=123, "Status 10 Frame Rate"=124, "Current Limit Threshold"=125, "CustomParam0"=137, "CustomParam1"=138, "PersStorageSaving"=139, "ClearPositionOnLimitF"=144, "ClearPositionOnLimitR"=145, "NominalBatteryVoltage"=146, "SampleVelocityPeriod"=147, "SampleVelocityWindow"=148] ("Parameter")
          w444 = T10 77 items=["Slot 0 - P"=1, "Slot 0 - I"=2, "Slot 0 - D"=3, "Slot 0 - F"=4, "Slot 0 - I Zone"=5, "Slot 0 - Ramp Rate"=6, "Slot 1 - P"=11, "Slot 1 - I"=12, "Slot 1 - D"=13, "Slot 1 - F"=14, "Slot 1 - I Zone"=15, "Slot 1 - Ramp Rate"=16, "Soft Limit - Forward"=21, "Soft Limit - Reverse"=22, "Soft Limit - Forward Enable"=23, "Soft Limit - Reverse Enable"=24, "On Boot - Brake Mode"=31, "On Boot - Limit Normally Closed - Forward"=32, "On Boot - Limit Normally Closed - Reverse"=33, "On Boot - Limit Disabled - Forward"=34, "On Boot - Limit Disabled - Reverse"=35, "Fault - Over Temp"=41, "Fault - Under Voltage"=42, "Fault - Forward Limit"=43, "Fault - Reverse Limit"=44, "Fault - Hardware Failure"=45, "Fault - Forward Soft Limit"=46, "Fault - Reverse Soft Limit"=47, "Sticky Fault - Over Temp"=48, "Sticky Fault - Under Voltage"=49, "Sticky Fault - Forward Limit"=50, "Sticky Fault - Reverse Limit"=51, "Sticky Fault - Forward Soft Limit"=52, "Sticky Fault - Reverse Soft Limit"=53, "Applied Throttle"=61, "Closed-Loop Error"=62, "Select Feedback Device"=63, "Reverse Closed-Loop Output"=64, "Mode Select"=65, "Profile Slot Select"=66, "Ramp Throttle"=67, "Reverse Feedback Sensor"=68, "Limit Switch Enabled"=69, "Limit Switch Closed - Forward"=70, "Limit Switch Closed - Reverse"=71, "Sensor Position"=73, "Sensor Velocity"=74, "Current"=75, "Brake is Enabled"=76, "Encoder Position"=77, "Encoder Velocity"=78, "Encoder Index Rise Events"=79, "Encoder A Pin State"=80, "Encoder B Pin State"=81, "Encoder Index Pin State"=82, "Analog In with Overflow"=83, "Analog In Velocity"=84, "Temperature"=85, "Battery Voltage"=86, "Reset Count"=87, "Reset Flags"=88, "Firmware Version"=89, "Settings Changed"=90, "Quad Filter Enable"=91, "Ignore Disable Broadcast"=92, "I Accumulator"=93, "Status 1 Frame Rate Ms"=94, "Status 2 Frame Rate Ms"=95, "Status 3 Frame Rate Ms"=96, "Status 4 Frame Rate Ms"=97, "Status 6 Frame Rate Ms"=98, "Status 7 Frame Rate Ms"=99, "Enable Index Pin Clear Position"=100, "Peak Positive Output"=104, "Nominal Positive Output"=105, "Peak Negative Output"=106, "Nominal Negative Output"=107, "Quad Index Pin Polarity"=108, "Status 8 Frame Rate Ms"=109, "Allow Position Overflow"=110, "Slot 0 - Allowable Closed-Loop Error"=111, "Number Potentiometer Turns"=112, "Encoder Codes Per Rev"=113, "Pulse Width Decoded Position"=114, "Analog Position"=115, "Voltage Compensation Rate (V/s)"=116, "Slot 1 - Allowable Closed-Loop Error"=117, "Motion Profile Has Underrun Err"=119, "Reserved 120"=120, "Legacy Control Mode"=121, "Motion Magic Acceleration"=122, "Motion Magic Cruise Velocity"=123, "Status 10 Frame Rate"=124, "Current Limit Threshold"=125, "CustomParam0"=137, "CustomParam1"=138, "PersStorageSaving"=139, "ClearPositionOnLimitF"=144, "ClearPositionOnLimitR"=145, "NominalBatteryVoltage"=146, "SampleVelocityPeriod"=147, "SampleVelocityWindow"=148] ("Parameter")
          n168 = Unbundle By Name(w442) -> ("CAN.Device Number"=w448:u8)
          n169 = Unbundle By Name(w441) -> ("CAN.Device Number"=w443:u8)
          n170 = call <vilib>:"WPI_CANTalonSRX_SetParameter.vi"("Value"=0.0, "Parameter"=w447, "Device ID (0)"=w448) -> ()  [unwired: 7 in, 2 out]
          n171 = call <vilib>:"WPI_CANTalonSRX_SetParameter.vi"("Value"=0.0, "Parameter"=w444, "Device ID (0)"=w443) -> ()  [unwired: 7 in, 2 out]
        }
        frame #5 {
          n172 = while {
            tunnel: w451 -> [w459]
            tunnel: [w452] -> w449
            stop <- w453 stop-if-true
            n173 = call <vilib>:"WPI_CANTalonSRX_GetStatus.vi"("CAN Talon SRX Ref"=w459) -> ("Talon SRX Status"=w458:T11, "CAN Talon SRX Ref"=w454:T4)  [unwired: 8 in, 1 out]
            n174 = Unbundle By Name(w458) -> ("Encoder Position"=w457:dbl)
            n175 = Less?(x=-1500.0, y=w457) -> (x < y?=w453:bool)
            n176 = case shown="False" w453 {
              tunnel: [-0.3 ("Output") 0.0 ("Output")] -> w455
              frame False {
              }
              frame True {
              }
            }
            n177 = call <vilib>:"WPI_MotorControlSetOutput.vi"("Output"=w455, "MotorControlDevRef"=w454) -> ("MotorControlDevRef"=w452:T4)  [unwired: 7 in, 2 out]
          }
        }
        frame #6 {
          w464 = T10 77 items=["Slot 0 - P"=1, "Slot 0 - I"=2, "Slot 0 - D"=3, "Slot 0 - F"=4, "Slot 0 - I Zone"=5, "Slot 0 - Ramp Rate"=6, "Slot 1 - P"=11, "Slot 1 - I"=12, "Slot 1 - D"=13, "Slot 1 - F"=14, "Slot 1 - I Zone"=15, "Slot 1 - Ramp Rate"=16, "Soft Limit - Forward"=21, "Soft Limit - Reverse"=22, "Soft Limit - Forward Enable"=23, "Soft Limit - Reverse Enable"=24, "On Boot - Brake Mode"=31, "On Boot - Limit Normally Closed - Forward"=32, "On Boot - Limit Normally Closed - Reverse"=33, "On Boot - Limit Disabled - Forward"=34, "On Boot - Limit Disabled - Reverse"=35, "Fault - Over Temp"=41, "Fault - Under Voltage"=42, "Fault - Forward Limit"=43, "Fault - Reverse Limit"=44, "Fault - Hardware Failure"=45, "Fault - Forward Soft Limit"=46, "Fault - Reverse Soft Limit"=47, "Sticky Fault - Over Temp"=48, "Sticky Fault - Under Voltage"=49, "Sticky Fault - Forward Limit"=50, "Sticky Fault - Reverse Limit"=51, "Sticky Fault - Forward Soft Limit"=52, "Sticky Fault - Reverse Soft Limit"=53, "Applied Throttle"=61, "Closed-Loop Error"=62, "Select Feedback Device"=63, "Reverse Closed-Loop Output"=64, "Mode Select"=65, "Profile Slot Select"=66, "Ramp Throttle"=67, "Reverse Feedback Sensor"=68, "Limit Switch Enabled"=69, "Limit Switch Closed - Forward"=70, "Limit Switch Closed - Reverse"=71, "Sensor Position"=73, "Sensor Velocity"=74, "Current"=75, "Brake is Enabled"=76, "Encoder Position"=77, "Encoder Velocity"=78, "Encoder Index Rise Events"=79, "Encoder A Pin State"=80, "Encoder B Pin State"=81, "Encoder Index Pin State"=82, "Analog In with Overflow"=83, "Analog In Velocity"=84, "Temperature"=85, "Battery Voltage"=86, "Reset Count"=87, "Reset Flags"=88, "Firmware Version"=89, "Settings Changed"=90, "Quad Filter Enable"=91, "Ignore Disable Broadcast"=92, "I Accumulator"=93, "Status 1 Frame Rate Ms"=94, "Status 2 Frame Rate Ms"=95, "Status 3 Frame Rate Ms"=96, "Status 4 Frame Rate Ms"=97, "Status 6 Frame Rate Ms"=98, "Status 7 Frame Rate Ms"=99, "Enable Index Pin Clear Position"=100, "Peak Positive Output"=104, "Nominal Positive Output"=105, "Peak Negative Output"=106, "Nominal Negative Output"=107, "Quad Index Pin Polarity"=108, "Status 8 Frame Rate Ms"=109, "Allow Position Overflow"=110, "Slot 0 - Allowable Closed-Loop Error"=111, "Number Potentiometer Turns"=112, "Encoder Codes Per Rev"=113, "Pulse Width Decoded Position"=114, "Analog Position"=115, "Voltage Compensation Rate (V/s)"=116, "Slot 1 - Allowable Closed-Loop Error"=117, "Motion Profile Has Underrun Err"=119, "Reserved 120"=120, "Legacy Control Mode"=121, "Motion Magic Acceleration"=122, "Motion Magic Cruise Velocity"=123, "Status 10 Frame Rate"=124, "Current Limit Threshold"=125, "CustomParam0"=137, "CustomParam1"=138, "PersStorageSaving"=139, "ClearPositionOnLimitF"=144, "ClearPositionOnLimitR"=145, "NominalBatteryVoltage"=146, "SampleVelocityPeriod"=147, "SampleVelocityWindow"=148] ("Parameter")
          w468 = T10 77 items=["Slot 0 - P"=1, "Slot 0 - I"=2, "Slot 0 - D"=3, "Slot 0 - F"=4, "Slot 0 - I Zone"=5, "Slot 0 - Ramp Rate"=6, "Slot 1 - P"=11, "Slot 1 - I"=12, "Slot 1 - D"=13, "Slot 1 - F"=14, "Slot 1 - I Zone"=15, "Slot 1 - Ramp Rate"=16, "Soft Limit - Forward"=21, "Soft Limit - Reverse"=22, "Soft Limit - Forward Enable"=23, "Soft Limit - Reverse Enable"=24, "On Boot - Brake Mode"=31, "On Boot - Limit Normally Closed - Forward"=32, "On Boot - Limit Normally Closed - Reverse"=33, "On Boot - Limit Disabled - Forward"=34, "On Boot - Limit Disabled - Reverse"=35, "Fault - Over Temp"=41, "Fault - Under Voltage"=42, "Fault - Forward Limit"=43, "Fault - Reverse Limit"=44, "Fault - Hardware Failure"=45, "Fault - Forward Soft Limit"=46, "Fault - Reverse Soft Limit"=47, "Sticky Fault - Over Temp"=48, "Sticky Fault - Under Voltage"=49, "Sticky Fault - Forward Limit"=50, "Sticky Fault - Reverse Limit"=51, "Sticky Fault - Forward Soft Limit"=52, "Sticky Fault - Reverse Soft Limit"=53, "Applied Throttle"=61, "Closed-Loop Error"=62, "Select Feedback Device"=63, "Reverse Closed-Loop Output"=64, "Mode Select"=65, "Profile Slot Select"=66, "Ramp Throttle"=67, "Reverse Feedback Sensor"=68, "Limit Switch Enabled"=69, "Limit Switch Closed - Forward"=70, "Limit Switch Closed - Reverse"=71, "Sensor Position"=73, "Sensor Velocity"=74, "Current"=75, "Brake is Enabled"=76, "Encoder Position"=77, "Encoder Velocity"=78, "Encoder Index Rise Events"=79, "Encoder A Pin State"=80, "Encoder B Pin State"=81, "Encoder Index Pin State"=82, "Analog In with Overflow"=83, "Analog In Velocity"=84, "Temperature"=85, "Battery Voltage"=86, "Reset Count"=87, "Reset Flags"=88, "Firmware Version"=89, "Settings Changed"=90, "Quad Filter Enable"=91, "Ignore Disable Broadcast"=92, "I Accumulator"=93, "Status 1 Frame Rate Ms"=94, "Status 2 Frame Rate Ms"=95, "Status 3 Frame Rate Ms"=96, "Status 4 Frame Rate Ms"=97, "Status 6 Frame Rate Ms"=98, "Status 7 Frame Rate Ms"=99, "Enable Index Pin Clear Position"=100, "Peak Positive Output"=104, "Nominal Positive Output"=105, "Peak Negative Output"=106, "Nominal Negative Output"=107, "Quad Index Pin Polarity"=108, "Status 8 Frame Rate Ms"=109, "Allow Position Overflow"=110, "Slot 0 - Allowable Closed-Loop Error"=111, "Number Potentiometer Turns"=112, "Encoder Codes Per Rev"=113, "Pulse Width Decoded Position"=114, "Analog Position"=115, "Voltage Compensation Rate (V/s)"=116, "Slot 1 - Allowable Closed-Loop Error"=117, "Motion Profile Has Underrun Err"=119, "Reserved 120"=120, "Legacy Control Mode"=121, "Motion Magic Acceleration"=122, "Motion Magic Cruise Velocity"=123, "Status 10 Frame Rate"=124, "Current Limit Threshold"=125, "CustomParam0"=137, "CustomParam1"=138, "PersStorageSaving"=139, "ClearPositionOnLimitF"=144, "ClearPositionOnLimitR"=145, "NominalBatteryVoltage"=146, "SampleVelocityPeriod"=147, "SampleVelocityWindow"=148] ("Parameter")
          n178 = Unbundle By Name(w466) -> ("CAN.Device Number"=w467:u8)
          n179 = Unbundle By Name(w462) -> ("CAN.Device Number"=w465:u8)
          n180 = call <vilib>:"WPI_CANTalonSRX_SetParameter.vi"("Value"=0.0, "Parameter"=w468, "Device ID (0)"=w467) -> ()  [unwired: 7 in, 2 out]
          n181 = call <vilib>:"WPI_CANTalonSRX_SetParameter.vi"("Value"=0.0, "Parameter"=w464, "Device ID (0)"=w465) -> ()  [unwired: 7 in, 2 out]
        }
        frame #7 {
          n182 = while {
            tunnel: w473 -> [w490]
            tunnel: w472 -> [w479]
            tunnel: [w475] -> w471
            tunnel: [w474] -> w470
            stop <- w476 stop-if-true
            n183 = call <vilib>:"WPI_CANTalonSRX_GetStatus.vi"("CAN Talon SRX Ref"=w490) -> ("Talon SRX Status"=w489:T11, "CAN Talon SRX Ref"=w488:T4)  [unwired: 8 in, 1 out]
            n184 = call <vilib>:"WPI_CANTalonSRX_GetStatus.vi"("CAN Talon SRX Ref"=w479) -> ("Talon SRX Status"=w480:T11, "CAN Talon SRX Ref"=w481:T4)  [unwired: 8 in, 1 out]
            n185 = Unbundle By Name(w489) -> ("Encoder Position"=w487:dbl)
            n186 = Unbundle By Name(w480) -> ("Encoder Position"=w482:dbl)
            n187 = Less?(x=-4500.0, y=w487) -> (x < y?=w477:bool)
            n188 = Greater?(x=9375.0, y=w482) -> (0:w478:bool)
            n189 = case shown="False" w477 {
              tunnel: [-0.3 ("Output") 0.0 ("Output")] -> w485
              frame False {
              }
              frame True {
              }
            }
            n190 = case shown="False" w478 {
              tunnel: [-0.3 ("Output") 0.0 ("Output")] -> w484
              frame False {
              }
              frame True {
              }
            }
            n191 = And(x=w477, y=w478) -> (x .and. y?=w476:bool)
            n192 = call <vilib>:"WPI_MotorControlSetOutput.vi"("Output"=w485, "MotorControlDevRef"=w488) -> ("MotorControlDevRef"=w474:T4)  [unwired: 7 in, 2 out]
            n193 = call <vilib>:"WPI_MotorControlSetOutput.vi"("Output"=w484, "MotorControlDevRef"=w481) -> ("MotorControlDevRef"=w475:T4)  [unwired: 7 in, 2 out]
          }
        }
        frame #8 {
          w500 = T10 77 items=["Slot 0 - P"=1, "Slot 0 - I"=2, "Slot 0 - D"=3, "Slot 0 - F"=4, "Slot 0 - I Zone"=5, "Slot 0 - Ramp Rate"=6, "Slot 1 - P"=11, "Slot 1 - I"=12, "Slot 1 - D"=13, "Slot 1 - F"=14, "Slot 1 - I Zone"=15, "Slot 1 - Ramp Rate"=16, "Soft Limit - Forward"=21, "Soft Limit - Reverse"=22, "Soft Limit - Forward Enable"=23, "Soft Limit - Reverse Enable"=24, "On Boot - Brake Mode"=31, "On Boot - Limit Normally Closed - Forward"=32, "On Boot - Limit Normally Closed - Reverse"=33, "On Boot - Limit Disabled - Forward"=34, "On Boot - Limit Disabled - Reverse"=35, "Fault - Over Temp"=41, "Fault - Under Voltage"=42, "Fault - Forward Limit"=43, "Fault - Reverse Limit"=44, "Fault - Hardware Failure"=45, "Fault - Forward Soft Limit"=46, "Fault - Reverse Soft Limit"=47, "Sticky Fault - Over Temp"=48, "Sticky Fault - Under Voltage"=49, "Sticky Fault - Forward Limit"=50, "Sticky Fault - Reverse Limit"=51, "Sticky Fault - Forward Soft Limit"=52, "Sticky Fault - Reverse Soft Limit"=53, "Applied Throttle"=61, "Closed-Loop Error"=62, "Select Feedback Device"=63, "Reverse Closed-Loop Output"=64, "Mode Select"=65, "Profile Slot Select"=66, "Ramp Throttle"=67, "Reverse Feedback Sensor"=68, "Limit Switch Enabled"=69, "Limit Switch Closed - Forward"=70, "Limit Switch Closed - Reverse"=71, "Sensor Position"=73, "Sensor Velocity"=74, "Current"=75, "Brake is Enabled"=76, "Encoder Position"=77, "Encoder Velocity"=78, "Encoder Index Rise Events"=79, "Encoder A Pin State"=80, "Encoder B Pin State"=81, "Encoder Index Pin State"=82, "Analog In with Overflow"=83, "Analog In Velocity"=84, "Temperature"=85, "Battery Voltage"=86, "Reset Count"=87, "Reset Flags"=88, "Firmware Version"=89, "Settings Changed"=90, "Quad Filter Enable"=91, "Ignore Disable Broadcast"=92, "I Accumulator"=93, "Status 1 Frame Rate Ms"=94, "Status 2 Frame Rate Ms"=95, "Status 3 Frame Rate Ms"=96, "Status 4 Frame Rate Ms"=97, "Status 6 Frame Rate Ms"=98, "Status 7 Frame Rate Ms"=99, "Enable Index Pin Clear Position"=100, "Peak Positive Output"=104, "Nominal Positive Output"=105, "Peak Negative Output"=106, "Nominal Negative Output"=107, "Quad Index Pin Polarity"=108, "Status 8 Frame Rate Ms"=109, "Allow Position Overflow"=110, "Slot 0 - Allowable Closed-Loop Error"=111, "Number Potentiometer Turns"=112, "Encoder Codes Per Rev"=113, "Pulse Width Decoded Position"=114, "Analog Position"=115, "Voltage Compensation Rate (V/s)"=116, "Slot 1 - Allowable Closed-Loop Error"=117, "Motion Profile Has Underrun Err"=119, "Reserved 120"=120, "Legacy Control Mode"=121, "Motion Magic Acceleration"=122, "Motion Magic Cruise Velocity"=123, "Status 10 Frame Rate"=124, "Current Limit Threshold"=125, "CustomParam0"=137, "CustomParam1"=138, "PersStorageSaving"=139, "ClearPositionOnLimitF"=144, "ClearPositionOnLimitR"=145, "NominalBatteryVoltage"=146, "SampleVelocityPeriod"=147, "SampleVelocityWindow"=148] ("Parameter")
          w501 = T10 77 items=["Slot 0 - P"=1, "Slot 0 - I"=2, "Slot 0 - D"=3, "Slot 0 - F"=4, "Slot 0 - I Zone"=5, "Slot 0 - Ramp Rate"=6, "Slot 1 - P"=11, "Slot 1 - I"=12, "Slot 1 - D"=13, "Slot 1 - F"=14, "Slot 1 - I Zone"=15, "Slot 1 - Ramp Rate"=16, "Soft Limit - Forward"=21, "Soft Limit - Reverse"=22, "Soft Limit - Forward Enable"=23, "Soft Limit - Reverse Enable"=24, "On Boot - Brake Mode"=31, "On Boot - Limit Normally Closed - Forward"=32, "On Boot - Limit Normally Closed - Reverse"=33, "On Boot - Limit Disabled - Forward"=34, "On Boot - Limit Disabled - Reverse"=35, "Fault - Over Temp"=41, "Fault - Under Voltage"=42, "Fault - Forward Limit"=43, "Fault - Reverse Limit"=44, "Fault - Hardware Failure"=45, "Fault - Forward Soft Limit"=46, "Fault - Reverse Soft Limit"=47, "Sticky Fault - Over Temp"=48, "Sticky Fault - Under Voltage"=49, "Sticky Fault - Forward Limit"=50, "Sticky Fault - Reverse Limit"=51, "Sticky Fault - Forward Soft Limit"=52, "Sticky Fault - Reverse Soft Limit"=53, "Applied Throttle"=61, "Closed-Loop Error"=62, "Select Feedback Device"=63, "Reverse Closed-Loop Output"=64, "Mode Select"=65, "Profile Slot Select"=66, "Ramp Throttle"=67, "Reverse Feedback Sensor"=68, "Limit Switch Enabled"=69, "Limit Switch Closed - Forward"=70, "Limit Switch Closed - Reverse"=71, "Sensor Position"=73, "Sensor Velocity"=74, "Current"=75, "Brake is Enabled"=76, "Encoder Position"=77, "Encoder Velocity"=78, "Encoder Index Rise Events"=79, "Encoder A Pin State"=80, "Encoder B Pin State"=81, "Encoder Index Pin State"=82, "Analog In with Overflow"=83, "Analog In Velocity"=84, "Temperature"=85, "Battery Voltage"=86, "Reset Count"=87, "Reset Flags"=88, "Firmware Version"=89, "Settings Changed"=90, "Quad Filter Enable"=91, "Ignore Disable Broadcast"=92, "I Accumulator"=93, "Status 1 Frame Rate Ms"=94, "Status 2 Frame Rate Ms"=95, "Status 3 Frame Rate Ms"=96, "Status 4 Frame Rate Ms"=97, "Status 6 Frame Rate Ms"=98, "Status 7 Frame Rate Ms"=99, "Enable Index Pin Clear Position"=100, "Peak Positive Output"=104, "Nominal Positive Output"=105, "Peak Negative Output"=106, "Nominal Negative Output"=107, "Quad Index Pin Polarity"=108, "Status 8 Frame Rate Ms"=109, "Allow Position Overflow"=110, "Slot 0 - Allowable Closed-Loop Error"=111, "Number Potentiometer Turns"=112, "Encoder Codes Per Rev"=113, "Pulse Width Decoded Position"=114, "Analog Position"=115, "Voltage Compensation Rate (V/s)"=116, "Slot 1 - Allowable Closed-Loop Error"=117, "Motion Profile Has Underrun Err"=119, "Reserved 120"=120, "Legacy Control Mode"=121, "Motion Magic Acceleration"=122, "Motion Magic Cruise Velocity"=123, "Status 10 Frame Rate"=124, "Current Limit Threshold"=125, "CustomParam0"=137, "CustomParam1"=138, "PersStorageSaving"=139, "ClearPositionOnLimitF"=144, "ClearPositionOnLimitR"=145, "NominalBatteryVoltage"=146, "SampleVelocityPeriod"=147, "SampleVelocityWindow"=148] ("Parameter")
          n194 = Unbundle By Name(w498) -> ("CAN.Device Number"=w495:u8)
          n195 = Unbundle By Name(w496) -> ("CAN.Device Number"=w497:u8)
          n196 = call <vilib>:"WPI_CANTalonSRX_SetParameter.vi"("Value"=0.0, "Parameter"=w501, "Device ID (0)"=w495) -> ()  [unwired: 7 in, 2 out]
          n197 = call <vilib>:"WPI_CANTalonSRX_SetParameter.vi"("Value"=0.0, "Parameter"=w500, "Device ID (0)"=w497) -> ()  [unwired: 7 in, 2 out]
        }
      }
    }
    frame "Forward" {
      n198 = call-poly <vilib>:"WPI_RobotDriveArcadeDrive.vi"("error in (no error)"=w507, "Y axis value"=0.55, "RobotDriveDevRef"=w508) -> ("error out"=w503:errorcluster, "RobotDriveDevRef"=w505:T8)  [unwired: 6 in, 1 out]
      n199 = call <vilib>:"WPI_RobotDriveDelayAndUpdateSafety.vi"("error in (no error)"=w503, "Delay (s)"=2.8, "RobotDriveDevRef"=w505) -> ()  [unwired: 7 in, 2 out]
    }
    frame "GEAR DROP" {
      n200 = call-poly <vilib>:"WPI_RobotDriveArcadeDrive.vi"("error in (no error)"=w532, "Y axis value"=0.45, "RobotDriveDevRef"=w533) -> ("error out"=w529:errorcluster, "RobotDriveDevRef"=w530:T8)  [unwired: 6 in, 1 out]
      n201 = call <vilib>:"WPI_RobotDriveDelayAndUpdateSafety.vi"("error in (no error)"=w529, "Delay (s)"=2.4, "RobotDriveDevRef"=w530) -> ("error out"=w527:errorcluster, "RobotDriveDevRef 2"=w526:T8)  [unwired: 7 in]
      n202 = call-poly <vilib>:"WPI_RobotDriveArcadeDrive.vi"("error in (no error)"=w527, "Y axis value"=0.0, "RobotDriveDevRef"=w526) -> ("error out"=w523:errorcluster, "RobotDriveDevRef"=w524:T8)  [unwired: 6 in, 1 out]
      n203 = call <vilib>:"WPI_RobotDriveDelayAndUpdateSafety.vi"("error in (no error)"=w523, "Delay (s)"=0.5, "RobotDriveDevRef"=w524) -> ("error out"=w516:errorcluster, "RobotDriveDevRef 2"=w515:T8)  [unwired: 7 in]
      n204 = while {
        tunnel: w516 -> [w545]
        tunnel: [w542] -> w514
        tunnel: w513 -> [w541]
        tunnel: [w540] -> w512
        stop <- w543 stop-if-true
        n205 = global read "Robot Global Data.vi" "LOWER LIMIT"() -> (w543:bool)
        n206 = call <vilib>:"WPI_MotorControlSetOutput.vi"("error in (no error)"=w545, "Output"=-0.6 ("f"), "MotorControlDevRef"=w541) -> ("error out"=w542:errorcluster, "MotorControlDevRef"=w540:T4)  [unwired: 6 in, 1 out]
      }
      n207 = call-poly <vilib>:"WPI_RobotDriveArcadeDrive.vi"("error in (no error)"=w514, "Y axis value"=-0.4, "RobotDriveDevRef"=w515) -> ("error out"=w520:errorcluster, "RobotDriveDevRef"=w519:T8)  [unwired: 6 in, 1 out]
      n208 = call <vilib>:"WPI_RobotDriveDelayAndUpdateSafety.vi"("error in (no error)"=w520, "Delay (s)"=1.5, "RobotDriveDevRef"=w519) -> ("error out"=w511:errorcluster)  [unwired: 7 in, 1 out]
      n209 = while {
        tunnel: w512 -> [w538]
        tunnel: w511 -> [w536]
        tunnel: [w535] -> w510
        tunnel: [w534] -> w509
        stop <- w539 stop-if-true
        n210 = call <vilib>:"WPI_MotorControlSetOutput.vi"("error in (no error)"=w536, "Output"=0.6, "MotorControlDevRef"=w538) -> ("error out"=w534:errorcluster, "MotorControlDevRef"=w535:T4)  [unwired: 6 in, 1 out]
        n211 = global read "Robot Global Data.vi" "UPPER LIMIT"() -> (w539:bool)
      }
      n212 = call <vilib>:"WPI_MotorControlSetOutput.vi"("error in (no error)"=w509, "Output"=0.0, "MotorControlDevRef"=w510) -> ()  [unwired: 6 in, 3 out]
    }
  }
